vi "park snom main.vi"() -> ()   [LabVIEW 2021]
panel:
  in  "Comments 3":string
  in  "Comments 2":string
  in  "Comments 1":string
  in  "Load Pos 3":bool
  in  "Load Pos 2":bool
  in  "Load Pos 1":bool
  in  "Save Position 3":bool
  in  "Save Position 2":bool
  out "Position 3":T1
  out "Position 2":T1
  out "Position 1":T1
  in  "Time To Wait":dbl
  out "Scan Origin (ALS)":T1
  in  "minimum value":dbl=-5.0 format="%0.2f"
  in  "maximum value":dbl=5.0 format="%0.2f"
  in  "Read pos on/off":bool
  in  "Save Waveform Graph":bool
  in  "Update\nphi/theta":bool
  in  "dz":dbl
  in  "dy":dbl
  in  "dx":dbl
  in  "Move to rho":bool
  out "Current Volts":dbl format="%0.7f"
  out "Waveform Graph":dbl[](graph)
  in  "Angeled Line\nScan":bool
  in  "rho Step Size (microns)":dbl=10.0
  in  "rho Length (microns)":dbl=1000.0
  in  "phi":dbl
  in  "theta":dbl
  in  "Z":string="3"
  in  "Y":string="2"
  in  "X":string="1"
  in  "First Time?":bool
  in  "Save Position 1":bool
  out "Estimated\nTime Left":dbl
  out "Percent Complete":dbl
  in  "Back scan delay":u32
  in  "Angled Scan":bool
  in  "Angle":dbl
  out "Scan Type":string="Start Point Serpent Scan"
  in  "T=SP \nf=CP":bool
  in  "Save Intensity Graph":bool
  in  "Export Data to Excel":bool
  in  "Center Typewritter\nScan":bool
  in  "Center Serpent\nScan":bool
  out "Measured":dbl
  out "Absolute 1 time":u32
  in  "physical channels":tag="Dev1/ai7"
  out "Time per Pixel":u32
  in  "Command":string
  in  "Controller #":string
  in  "Command":bool
  out "Graph":dbl[][](graph)
  in  "rate":dbl=250000.0
  in  "number of samples":i32=100
  out "Slow Axis Pos\n(Max)":dbl
  out "Fast Axis Pos\n(Max)":dbl
  out "Min Value":dbl
  in  "Move to Max\nValue Position":bool
  out "Max Value":dbl
  in  "Move to Cursor 2":bool
  in  "Move to Cursor 1":bool
  out "Scan Origin":T1
  in  "Move 3 By":dbl=1.0
  in  "Move 2 By":dbl=1.0
  in  "Move 3 to":dbl=12.0
  in  "Move 2 to":dbl=3.8
  in  "PL 3":dbl=22.2
  in  "PL 2":dbl=12.2
  in  "PL 1":dbl=12.2
  in  "NL 3":dbl
  in  "NL 2":dbl
  in  "NL 1":dbl
  in  "Set Limits":bool
  in  "Move All":bool
  in  "Update Params":bool
  in  "Start Point\nTypewriter Scan":bool
  in  "Initialize?":bool
  in  "Abort Scan":bool
  in  "Start Point\nSerpent Scan":bool
  in  "Slow Length (microns)":dbl=500.0
  in  "Slow Step Size (microns)":dbl=100.0
  in  "Fast Length (microns)":dbl=500.0
  in  "Fast Step Size (microns)":dbl=100.0
  in  "Slow Axis":string="3"
  in  "Fast Axis":string="1"
  in  "Update Loop Type":bool
  in  "Loop Type":string="2"
  in  "Motion Parameters In":T2={"Velocity"=2.0, "Deceleration "=100.0, "Acceleration"=100.0}
  out "Motion Parameters Out":T3={"Velocity "=2.0, "Deceleration "=100.0, "Acceleration"=100.0}
  out "Calculated Position":T1
  out "Encoder Position":T4
  in  "Move 1 to":dbl=6.0
  in  "Move 1 By":dbl=1.0
  in  "Motor 3":bool
  in  "Motor 2":bool
  in  "< 3":bool
  in  "> 3":bool
  in  "< 2":bool
  in  "> 2":bool
  in  "<":bool
  in  ">":bool
  in  "Motor 1":bool
  in  "End":bool
  # "Positioning"
  # "Motion Parameters"
  # "mm/s"
  # "mm"
  # "mm"
  # "Controller #1"
  # "mm"
  # "mm/s^2"
  # "Controller #2"
  # "mm"
  # "mm"
  # "mm/s^2"
  # "Controller #3"
  # "mm"
  # "mm"
  # "mm"
  # "V"
  # "msec"
  # "Motor 1"
  # "mm"
  # "mm"
  # "min"
  # "Motor 2"
  # "0: Open Loop\n2: Clean Closed Loop\n3: Closed Loop"
  # "mm"
  # "mm"
  # "Motor 3"
  # "mm"
  # "mm"
  # "mm"
  # "mm"
  # "mm"
  # "mm"
  # "Might have to\npress twice"
  # "mm"
  # "mm"
  # "mm"
  # "mm"
  # "mm"
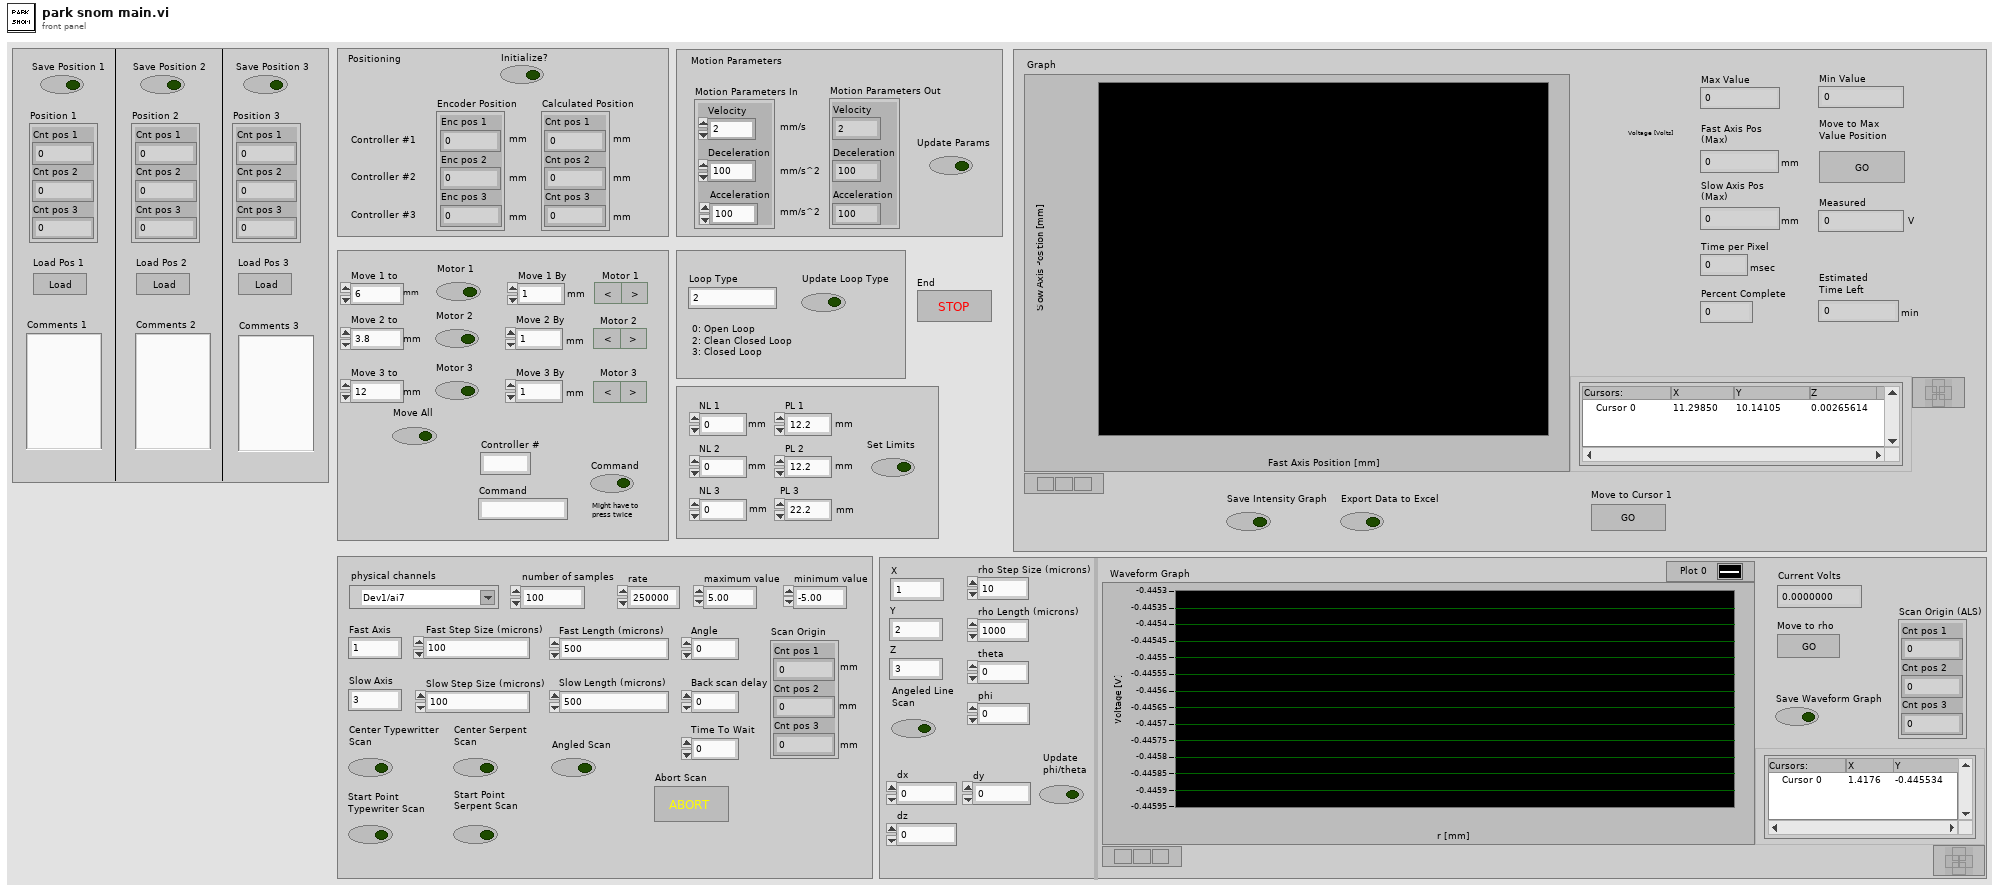
[diagram p1: front panel]
types:
  T1 = cluster{"Cnt pos 1":dbl, "Cnt pos 2":dbl, "Cnt pos 3":dbl}
  T2 = cluster{"Velocity":dbl, "Deceleration ":dbl, "Acceleration":dbl}
  T3 = cluster{"Velocity ":dbl, "Deceleration ":dbl, "Acceleration":dbl}
  T4 = cluster{"Enc pos 1":dbl, "Enc pos 2":dbl, "Enc pos 3":dbl}
  T5 = cluster{"P type":u16, "VISA resource name out":refnum<visa-resource-name>, " Terminator":string, "Timeout":i32}
  T6 = cluster{"P type":u16, "reference":refnum<visa-resource-name>, " Terminator ":string, "Timeout":i32}
  T7 = typedef "LVPointDoubleTypeDef.ctl" = cluster{"Cursor X":dbl, "Cursor Y":dbl}
  T8 = typedef "LVCursorListTypeDef.ctl" = cluster{"Name":string, "Color":u32, "Style":u8, "Point Style":u8, "Name Visible":bool, "Allow Drag":bool, "Cursor Mode":u32, "Plot":i32, "Index":i32, "Position":cluster{"X":dbl, "Y":dbl}, "X Scale":u32, "Y Scale":u32, "Watch Plots":i32[], "Watch All Plots":bool, "Plot Area":i32, "Label Offset":cluster{"X":dbl, "Y":dbl}}[]
  T9 = typedef "imagedata.ctl" = cluster{"image type":i32, "image depth":i32, "image":u8[], "mask":u8[], "colors":u32[], "Rectangle":cluster{"left":i16, "top":i16, "right":i16, "bottom":i16}}
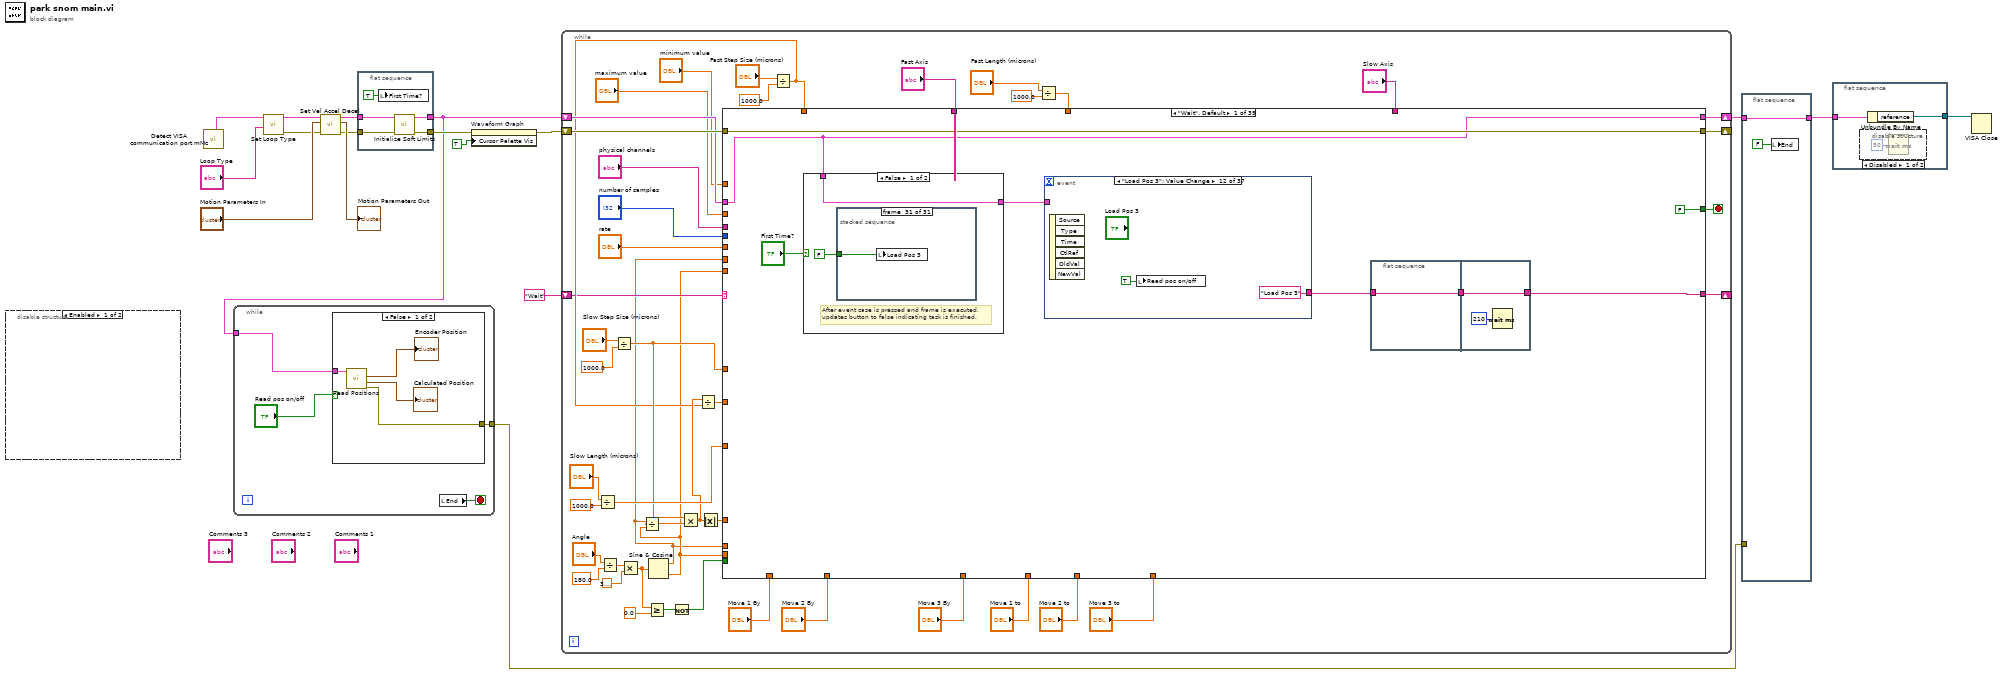
[diagram p0: block diagram]
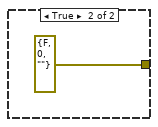
[diagram p2: hidden frame]
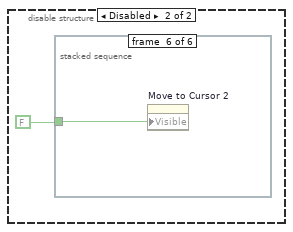
[diagram p3: hidden frame]
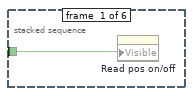
[diagram p4: hidden frame]
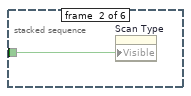
[diagram p5: hidden frame]
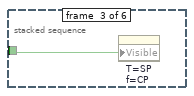
[diagram p6: hidden frame]
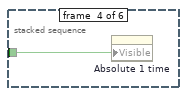
[diagram p7: hidden frame]
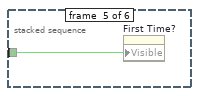
[diagram p8: hidden frame]
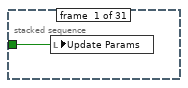
[diagram p10: hidden frame]
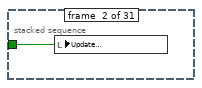
[diagram p11: hidden frame]
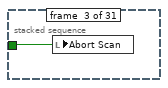
[diagram p12: hidden frame]
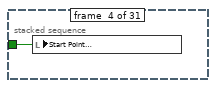
[diagram p13: hidden frame]
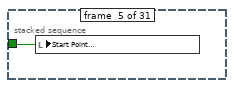
[diagram p14: hidden frame]
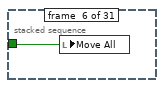
[diagram p15: hidden frame]
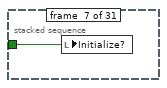
[diagram p16: hidden frame]
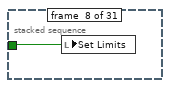
[diagram p17: hidden frame]
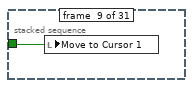
[diagram p18: hidden frame]
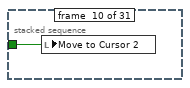
[diagram p19: hidden frame]
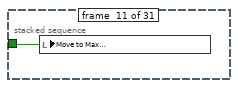
[diagram p20: hidden frame]
diagram:
  n1 = disable-structure shown="Enabled" {
    frame Enabled {
    }
    frame Disabled {
      n2 = stacked-sequence {
        tunnel: FALSE -> [w19 w20 w21 w22 w23 w24]
        frame #0 {
          n3 = property on="Read pos on/off" class="Bool (strict)"("Visible"=w19) -> ()  [unwired: 2 in, 2 out]
        }
        frame #1 {
          n4 = property on="Scan Type" class="Str"("Visible"=w20) -> ()  [unwired: 2 in, 2 out]
        }
        frame #2 {
          n5 = property on="T=SP \nf=CP" class="Bool (strict)"("Visible"=w21) -> ()  [unwired: 2 in, 2 out]
        }
        frame #3 {
          n6 = property on="Absolute 1 time" class="DigNum (strict)"("Visible"=w22) -> ()  [unwired: 2 in, 2 out]
        }
        frame #4 {
          n7 = property on="First Time?" class="Bool (strict)"("Visible"=w23) -> ()  [unwired: 2 in, 2 out]
        }
        frame #5 {
          n8 = property on="Move to Cursor 2" class="Bool (strict)"("Visible"=w24) -> ()  [unwired: 2 in, 2 out]
        }
      }
    }
  }
  n9 = call "Detect VISA communication port mMc.vi"() -> ("Port"=w14:T5)  [unwired: 6 in, 3 out]
  n10 = while {
    tunnel: w1 -> [w26]
    tunnel: [w27] -> w8
    stop <- w28 stop-if-true
    n11 = case shown="False" "Read pos on/off" {
      tunnel: [w30 errorcluster {"status"=FALSE, "code"=0, "source"=""} ("error out")] -> w27
      tunnel: w26 -> [w29 _]
      frame False {
        n12 = call "Read Positions.vi"("Port In"=w29) -> ("error out"=w30:errorcluster, "Calculated Position"=→"Calculated Position":T1, "Encoder Position"=→"Encoder Position":T4)  [unwired: 7 in, 1 out]
      }
      frame True {
      }
    }
    n13 = local read "End"() -> (w28:bool)
  }
  n14 = call "Set Loop Type.vi"("Loop Type"="Loop Type", "Port In"=w14) -> ("error out"=w5:errorcluster, "Port Out"=w12:T5)  [unwired: 8 in]
  n15 = call "Set Vel Accel Decel.vi"("error in (no error)"=w5, "Motion Parameters In"="Motion Parameters In", "Port In"=w12) -> ("error out"=w6:errorcluster, "Motion Parameters Out"=→"Motion Parameters Out":T3, "Port Out"=w7:T5)  [unwired: 6 in]
  n16 = flat-sequence {
    tunnel: w7 -> [w38]
    tunnel: w6 -> [w37]
    tunnel: [w36] -> w1
    tunnel: [w35] -> w3
    frame #0 {
      n17 = local write "First Time?"(TRUE ("first time")) -> ()
      n18 = call "Initialize Soft Limits.vi"("error in (no error)"=w37, "Port In"=w38) -> ("error out"=w35:errorcluster, "Port Out"=w36:T6)  [unwired: 8 in]
    }
  }
  n19 = property on="Waveform Graph" class="WFGraph (strict)"(error in=w3, "Cursor Palette Vis"=TRUE ("Cursor Legend Visible")) -> (error out=w2:errorcluster)  [unwired: 1 in, 1 out]
  n20 = while {
    shift-right: [w84] -> _
    shift-left: "Wait" -> [w48]
    shift-right: [w80] -> _
    shift-left: w2 -> [w83]
    shift-right: [w79] -> w10
    shift-left: w1 -> [w68]
    stop <- w81 stop-if-true
    n21 = Divide(x="Slow Length (microns)", y=1000.0) -> (x/y=w54:dbl)
    n22 = Divide(x="Angle", y=180.0) -> (x/y=w56:dbl)
    n23 = Divide(x="Slow Step Size (microns)", y=1000.0) -> (x/y=w51:dbl)
    n24 = Multiply(x=w56, y=3.141592653589793) -> (x*y=w44:dbl)
    n25 = Greater Or Equal?(x=w44, y=0.0) -> (x >= y?=w46:bool)
    n26 = Sine & Cosine(0:w44) -> (1:w41:dbl, 2:w42:dbl)
    n27 = Divide(x=w41, y=w42) -> (x/y=w43:dbl)
    n28 = Not(x=w46) -> (.not. x?=w45:bool)
    n29 = Multiply(x=w51, y=w43) -> (x*y=w50:dbl)
    n30 = Absolute Value(x=w50) -> (abs(x)=w53:dbl)
    n31 = Divide(x="Fast Step Size (microns)", y=1000.0) -> (x/y=w49:dbl)
    n32 = Divide(x=w50, y=w49) -> (x/y=w47:dbl)
    n33 = Divide(x="Fast Length (microns)", y=1000.0) -> (x/y=w60:dbl)
    n34 = case shown="\"Wait\", Default" w48 {
      tunnel: [w89 "Stop" "Update Limits" "Wait" "Wait" "Wait" "Wait" ("Scan Type") "Wait" ("Scan Type") "Wait" ("Scan Type") "Wait" ("Scan Type") "Wait" ("Scan Type") "Wait" ("Scan Type") "Wait" ("Scan Type") "Wait" "Wait" "Wait" "Wait" "Wait" "Wait" "Wait" "Wait" "Wait" "Wait" "Wait" w481 "Move to Origin" "Move to Origin" "Move to Origin" "Move to Origin" "Move to Origin" w1566 "Wait" "Wait" "Wait" "Wait" "Wait" ("Scan Type") "Wait" "Wait" "Wait"] -> w84
      tunnel: "Move 1 to" -> [_ _ _ _ _ _ _ _ _ _ _ _ _ w334 _ _ w384 _ _ _ _ _ _ _ _ _ _ _ _ _ _ _ _ _ _ _ _ _ _]
      tunnel: w68 -> [w85 w209 w218 w236 w248 w259 w264 w272 w277 w281 w289 w297 w315 w333 w359 w367 w379 w393 w411 w420 w429 w438 w447 w462 w483 w542 w732 w929 w1107 w1312 w1565 w1686 w1706 w1728 w1745 w1775 w1834 w1839 w1846]
      tunnel: w83 -> [w92 w211 w221 w235 w247 w257 w263 w271 w276 w282 w290 w298 w316 w342 w363 w371 w389 w397 w416 w425 w434 w443 w452 w463 w482 w552 w752 w940 w1140 w1341 w1592 w1683 w1703 w1723 w1740 w1782 w1837 w1840 w1847]
      tunnel: [w92 w211 w221 w233 w247 w257 w263 w271 w276 w282 w290 w298 w316 w342 w363 w371 w389 w397 w416 w425 w434 w443 w452 w463 w482 w552 w752 w940 w1140 w1341 w1592 w1683 w1703 w1723 w1740 w1782 w1837 w1840 w1847] -> w80
      tunnel: [FALSE TRUE FALSE FALSE FALSE FALSE FALSE FALSE FALSE FALSE FALSE FALSE FALSE FALSE FALSE FALSE FALSE FALSE FALSE FALSE FALSE FALSE FALSE FALSE FALSE FALSE FALSE FALSE FALSE FALSE FALSE FALSE FALSE FALSE FALSE FALSE FALSE FALSE FALSE] -> w81
      tunnel: [w85 w209 w222 w232 w244 w258 w264 w272 w277 w281 w289 w297 w315 w340 w357 w365 w373 w391 w409 w418 w427 w436 w445 w462 w483 w542 w732 w929 w1107 w1312 w1593 w1679 w1699 w1720 w1737 w1775 w1827 w1839 w1846] -> w79
      tunnel: w51 -> [_ _ _ _ _ _ _ _ _ _ _ _ _ _ _ _ _ _ _ _ _ _ _ _ w495 w546 w748 w935 w1136 w1337 _ _ _ _ _ _ _ _ _]
      tunnel: w54 -> [_ _ _ _ _ _ _ _ _ _ _ _ _ _ _ _ _ _ _ _ _ _ _ _ w485 w547 w738 w924 w1125 w1326 _ _ _ _ _ _ _ _ _]
      tunnel: w49 -> [_ _ _ _ _ _ _ _ _ _ _ _ _ _ _ _ _ _ _ _ _ _ _ _ w496 w531 w717 w920 w1100 w1311 _ _ _ _ _ _ _ _ _]
      tunnel: w60 -> [_ _ _ _ _ _ _ _ _ _ _ _ _ _ _ _ _ _ _ _ _ _ _ _ w493 w534 w719 w921 w1109 w1313 _ _ _ _ _ _ _ _ _]
      tunnel: "Fast Axis" -> [_ _ _ _ _ _ _ _ _ _ _ _ _ _ _ _ _ _ _ _ _ _ _ _ w494 w538 w726 w938 w1116 w1306 _ _ _ w1727 w1744 _ w1833 _ _]
      tunnel: "Slow Axis" -> [_ _ _ _ _ _ _ _ _ _ _ _ _ _ _ _ _ _ _ _ _ _ _ _ w486 w550 w730 w931 w1106 w1309 _ _ _ w1726 w1743 _ w1832 _ _]
      tunnel: "Move 2 to" -> [_ _ _ _ _ _ _ _ _ _ _ _ _ _ w358 _ w383 _ _ _ _ _ _ _ _ _ _ _ _ _ _ _ _ _ _ _ _ _ _]
      tunnel: "Move 3 to" -> [_ _ _ _ _ _ _ _ _ _ _ _ _ _ _ w366 w382 _ _ _ _ _ _ _ _ _ _ _ _ _ _ _ _ _ _ _ _ _ _]
      tunnel: "Move 1 By" -> [_ _ _ _ _ _ _ _ _ _ _ _ _ _ _ _ _ w392 _ _ w428 _ _ _ _ _ _ _ _ _ _ _ _ _ _ _ _ _ _]
      tunnel: "Move 2 By" -> [_ _ _ _ _ _ _ _ _ _ _ _ _ _ _ _ _ _ w410 _ _ w437 _ _ _ _ _ _ _ _ _ _ _ _ _ _ _ _ _]
      tunnel: "Move 3 By" -> [_ _ _ _ _ _ _ _ _ _ _ _ _ _ _ _ _ _ _ w419 _ _ w446 _ _ _ _ _ _ _ _ _ _ _ _ _ _ _ _]
      tunnel: "number of samples" -> [_ _ _ _ _ _ _ _ _ _ _ _ _ _ _ _ _ _ _ _ _ _ _ _ _ w537 w740 w925 w1128 w1329 w1568 _ _ _ _ _ _ _ _]
      tunnel: "rate" -> [_ _ _ _ _ _ _ _ _ _ _ _ _ _ _ _ _ _ _ _ _ _ _ _ _ w540 w742 w928 w1131 w1332 w1589 _ _ _ _ _ _ _ _]
      tunnel: "physical channels" -> [_ _ _ _ _ _ _ _ _ _ _ _ _ _ _ _ _ _ _ _ _ _ _ _ _ w539 w741 w926 w1129 w1330 w1590 _ _ _ _ _ _ _ _]
      tunnel: w53 -> [_ _ _ _ _ _ _ _ _ _ _ _ _ _ _ _ _ _ _ _ _ _ _ _ _ w532 w718 w919 w1101 _ _ _ _ _ _ _ _ _ _]
      tunnel: w45 -> [_ _ _ _ _ _ _ _ _ _ _ _ _ _ _ _ _ _ _ _ _ _ _ _ _ w535 w721 w922 w1111 _ _ _ _ _ _ _ _ _ _]
      tunnel: w47 -> [_ _ _ _ _ _ _ _ _ _ _ _ _ _ _ _ _ _ _ _ _ _ _ _ _ w525 w711 w913 w1110 _ _ _ _ _ _ _ _ _ _]
      tunnel: w42 -> [_ _ _ _ _ _ _ _ _ _ _ _ _ _ _ _ _ _ _ _ _ _ _ _ _ _ _ _ _ w1308 _ _ _ _ _ _ _ _ _]
      tunnel: w41 -> [_ _ _ _ _ _ _ _ _ _ _ _ _ _ _ _ _ _ _ _ _ _ _ _ _ _ _ _ _ w1307 _ _ _ _ _ _ _ _ _]
      tunnel: w42 -> [_ _ _ _ _ _ _ _ _ _ _ _ _ _ _ _ _ _ _ _ _ _ _ _ _ _ _ _ _ w1305 _ _ _ _ _ _ _ _ _]
      tunnel: w41 -> [_ _ _ _ _ _ _ _ _ _ _ _ _ _ _ _ _ _ _ _ _ _ _ _ _ _ _ _ _ w1304 _ _ _ _ _ _ _ _ _]
      tunnel: "maximum value" -> [_ _ _ _ _ _ _ _ _ _ _ _ _ _ _ _ _ _ _ _ _ _ _ _ _ w522 w709 w910 w1097 w1301 w1539 _ _ _ _ _ _ _ _]
      tunnel: "minimum value" -> [_ _ _ _ _ _ _ _ _ _ _ _ _ _ _ _ _ _ _ _ _ _ _ _ _ w521 w708 w909 w1096 w1300 w1538 _ _ _ _ _ _ _ _]
      frame "Wait", Default {
        n35 = case shown="False" "First Time?" {
          tunnel: [w93 w126] -> w86
          tunnel: w85 -> [w93 w126]
          frame False {
            # "After event case is pressed and frame is executed, \nupdates button to false indicating task is finished."
            n36 = stacked-sequence {
              tunnel: FALSE ("Command") -> [w95 w96 w97 w98 w99 w100 w101 w102 w103 w104 w105 w106 w107 w108 w109 w110 w111 w112 w113 w114 w115 w116 w117 w118 w119 w120 w121 w122 w123 w124 w125]
              frame #0 {
                n37 = local write "Update Params"(w95) -> ()
              }
              frame #1 {
                n38 = local write "Update\nphi/theta"(w96) -> ()
              }
              frame #2 {
                n39 = local write "Abort Scan"(w97) -> ()
              }
              frame #3 {
                n40 = local write "Start Point\nSerpent Scan"(w98) -> ()
              }
              frame #4 {
                n41 = local write "Start Point\nTypewriter Scan"(w99) -> ()
              }
              frame #5 {
                n42 = local write "Move All"(w100) -> ()
              }
              frame #6 {
                n43 = local write "Initialize?"(w101) -> ()
              }
              frame #7 {
                n44 = local write "Set Limits"(w102) -> ()
              }
              frame #8 {
                n45 = local write "Move to Cursor 1"(w103) -> ()
              }
              frame #9 {
                n46 = local write "Move to Cursor 2"(w104) -> ()
              }
              frame #10 {
                n47 = local write "Move to Max\nValue Position"(w105) -> ()
              }
              frame #11 {
                n48 = local write "Motor 1"(w106) -> ()
              }
              frame #12 {
                n49 = local write "Motor 2"(w107) -> ()
              }
              frame #13 {
                n50 = local write "Motor 3"(w108) -> ()
              }
              frame #14 {
                n51 = local write "Command"(w109) -> ()
              }
              frame #15 {
                n52 = local write "Center Serpent\nScan"(w110) -> ()
              }
              frame #16 {
                n53 = local write "Center Typewritter\nScan"(w111) -> ()
              }
              frame #17 {
                n54 = local write "Export Data to Excel"(w112) -> ()
              }
              frame #18 {
                n55 = local write "Save Intensity Graph"(w113) -> ()
              }
              frame #19 {
                n56 = local write "Angled Scan"(w114) -> ()
              }
              frame #20 {
                n57 = local write "Save Position 1"(w115) -> ()
              }
              frame #21 {
                n58 = local write "Angeled Line\nScan"(w116) -> ()
              }
              frame #22 {
                n59 = local write "Move to rho"(w117) -> ()
              }
              frame #23 {
                n60 = local write "Save Waveform Graph"(w118) -> ()
              }
              frame #24 {
                n61 = local write "Read pos on/off"(w119) -> ()
              }
              frame #25 {
                n62 = local write "Save Position 1"(w120) -> ()
              }
              frame #26 {
                n63 = local write "Save Position 2"(w121) -> ()
              }
              frame #27 {
                n64 = local write "Save Position 3"(w122) -> ()
              }
              frame #28 {
                n65 = local write "Load Pos 1"(w123) -> ()
              }
              frame #29 {
                n66 = local write "Load Pos 2"(w124) -> ()
              }
              frame #30 {
                n67 = local write "Load Pos 3"(w125) -> ()
              }
            }
          }
          frame True {
            n68 = local write "First Time?"(FALSE ("first time")) -> ()
          }
        }
        n69 = event shown="[11] \"Load Pos 3\": Value Change" {
          selector: _ -> [_ _ _ _ _ _ _ _ _ _ _ _ _ _ _ _ _ _ _ _ _ _ _ _ _ _ _ _ _ _ _ _ _ _ _ _ _]
          dyn-events: _ -> [_ _ _ _ _ _ _ _ _ _ _ _ _ _ _ _ _ _ _ _ _ _ _ _ _ _ _ _ _ _ _ _ _ _ _ _ _]
          timeout: _ -> [_ _ _ _ _ _ _ _ _ _ _ _ _ _ _ _ _ _ _ _ _ _ _ _ _ _ _ _ _ _ _ _ _ _ _ _ _]
          tunnel: ["Wait" "Stop" "Initialize" "Move Command" "Update Loop Type" "Update Params" "Save Position 1" "Save Position 2" "Save Position 3" "Load Pos 1" "Load Pos 2" "Load Pos 3" "Update phi/theta" "Motor 1 Absolute" "Motor 2 Absolute" "Motor 3 Absolute" "All Motors Absolute" "Motor 1 Positive Relative" "Motor 1 Negative Relative" "Motor 2 Positive Relative" "Motor 2 Negative Relative" "Motor 3 Positive Relative" "Motor 3 Negative Relative" "Update Limits" "Initialize Graph" "Initialize Graph" "Initialize Graph" "Initialize Graph" "Initialize Graph" "Angeled Line Scan" "Move to Cursor 1" "Move to Cursor 2" "Move to rho" "Move to Max Value Position" "Export Data" "Save Image" "Save Image"] -> w91
          tunnel: w86 -> [_ _ _ _ _ _ _ _ _ _ _ _ _ _ _ _ _ _ _ _ _ _ _ _ w169 w179 w182 w191 w197 w200 _ _ _ _ _ _ _]
          event Timeout {
            n70 = event-data() -> ()  [unwired: 1 in, 3 out]
          }
          event "End": Value Change {
            n71 = event-data() -> ()  [unwired: 1 in, 6 out]
          }
          event "Initialize?": Value Change {
            n72 = event-data() -> ()  [unwired: 1 in, 6 out]
          }
          event "Command": Value Change {
            n73 = event-data() -> ()  [unwired: 1 in, 6 out]
            n74 = local write "Command"(TRUE ("Command")) -> ()
          }
          event "Update Loop Type": Value Change {
            n75 = event-data() -> ()  [unwired: 1 in, 6 out]
          }
          event "Update Params": Value Change {
            n76 = event-data() -> ()  [unwired: 1 in, 6 out]
          }
          event "Save Position 1": Value Change {
            n77 = event-data() -> ()  [unwired: 1 in, 6 out]
            n78 = local write "Read pos on/off"(TRUE ("Save Position")) -> ()
          }
          event "Save Position 2": Value Change {
            n79 = event-data() -> ()  [unwired: 1 in, 6 out]
            n80 = local write "Read pos on/off"(TRUE ("Read pos on/off")) -> ()
          }
          event "Save Position 3": Value Change {
            n81 = event-data() -> ()  [unwired: 1 in, 6 out]
            n82 = local write "Read pos on/off"(TRUE ("Read pos on/off")) -> ()
          }
          event "Load Pos 1": Value Change {
            n83 = event-data() -> ()  [unwired: 1 in, 6 out]
            n84 = local write "Read pos on/off"(TRUE ("Read pos on/off")) -> ()
          }
          event "Load Pos 2": Value Change {
            n85 = event-data() -> ()  [unwired: 1 in, 6 out]
            n86 = local write "Read pos on/off"(TRUE ("Read pos on/off")) -> ()
          }
          event "Load Pos 3": Value Change {
            n87 = event-data() -> ()  [unwired: 1 in, 6 out]
            n88 = local write "Read pos on/off"(TRUE ("Read pos on/off")) -> ()
          }
          event "Update\nphi/theta": Value Change {
            n89 = event-data() -> ()  [unwired: 1 in, 6 out]
          }
          event "Motor 1": Value Change {
            n90 = event-data() -> ()  [unwired: 1 in, 6 out]
          }
          event "Motor 2": Value Change {
            n91 = event-data() -> ()  [unwired: 1 in, 6 out]
          }
          event "Motor 3": Value Change {
            n92 = event-data() -> ()  [unwired: 1 in, 6 out]
          }
          event "Move All": Value Change {
            n93 = event-data() -> ()  [unwired: 1 in, 6 out]
          }
          event ">": Value Change {
            n94 = event-data() -> ()  [unwired: 1 in, 6 out]
            n95 = local write "Read pos on/off"(TRUE ("Read pos on/off")) -> ()
          }
          event "<": Value Change {
            n96 = event-data() -> ()  [unwired: 1 in, 6 out]
            n97 = local write "Read pos on/off"(TRUE) -> ()
          }
          event "> 2": Value Change {
            n98 = event-data() -> ()  [unwired: 1 in, 6 out]
            n99 = local write "Read pos on/off"(TRUE) -> ()
          }
          event "< 2": Value Change {
            n100 = event-data() -> ()  [unwired: 1 in, 6 out]
            n101 = local write "Read pos on/off"(TRUE) -> ()
          }
          event "> 3": Value Change {
            n102 = event-data() -> ()  [unwired: 1 in, 6 out]
            n103 = local write "Read pos on/off"(TRUE) -> ()
          }
          event "< 3": Value Change {
            n104 = event-data() -> ()  [unwired: 1 in, 6 out]
            n105 = local write "Read pos on/off"(TRUE) -> ()
          }
          event "Set Limits": Value Change {
            n106 = event-data() -> ()  [unwired: 1 in, 6 out]
          }
          event "Start Point\nSerpent Scan": Value Change {
            n107 = event-data() -> ()  [unwired: 1 in, 6 out]
            n108 = local write "Read pos on/off"(TRUE ("Read pos on/off")) -> ()
            n109 = call "Read Positions.vi"("Port In"=w169) -> ("Calculated Position"=w173:T1)  [unwired: 7 in, 3 out]
            n110 = local write "Scan Origin"(w173) -> ()
            n111 = local write "T=SP \nf=CP"(TRUE ("T=SP \nf=CP")) -> ()
            "Scan Type" <- "Start Point Serpent Scan"
          }
          event "Center Serpent\nScan": Value Change {
            n112 = event-data() -> ()  [unwired: 1 in, 6 out]
            n113 = local write "Read pos on/off"(TRUE ("Read pos on/off")) -> ()
            n114 = local write "Scan Type"("Center Serpent Scan") -> ()
            n115 = call "Read Positions.vi"("Port In"=w179) -> ("Calculated Position"=w174:T1)  [unwired: 7 in, 3 out]
            n116 = local write "Scan Origin"(w174) -> ()
            n117 = local write "T=SP \nf=CP"(FALSE ("T=SP \nf=CP")) -> ()
          }
          event "Start Point\nTypewriter Scan": Value Change {
            n118 = event-data() -> ()  [unwired: 1 in, 6 out]
            n119 = local write "Read pos on/off"(TRUE ("Read pos on/off")) -> ()
            n120 = call "Read Positions.vi"("Port In"=w182) -> ("Calculated Position"=w185:T1)  [unwired: 7 in, 3 out]
            n121 = local write "Scan Type"("Start Point Typewriter Scan") -> ()
            n122 = local write "T=SP \nf=CP"(TRUE ("Status Bit")) -> ()
            n123 = local write "Scan Origin"(w185) -> ()
          }
          event "Center Typewritter\nScan": Value Change {
            n124 = event-data() -> ()  [unwired: 1 in, 6 out]
            n125 = local write "Read pos on/off"(TRUE ("Read pos on/off")) -> ()
            n126 = local write "Scan Type"("Center Typewriter Scan") -> ()
            n127 = call "Read Positions.vi"("Port In"=w191) -> ("Calculated Position"=w190:T1)  [unwired: 7 in, 3 out]
            n128 = local write "Scan Origin"(w190) -> ()
            n129 = local write "T=SP \nf=CP"(FALSE ("T=SP \nf=CP")) -> ()
          }
          event "Angled Scan": Value Change {
            n130 = event-data() -> ()  [unwired: 1 in, 6 out]
            n131 = local write "Read pos on/off"(TRUE ("Read pos on/off")) -> ()
            n132 = local write "Scan Type"("Angeled Scan") -> ()
            n133 = call "Read Positions.vi"("Port In"=w197) -> ("Calculated Position"=w196:T1)  [unwired: 7 in, 3 out]
            n134 = local write "Scan Origin"(w196) -> ()
            n135 = local write "T=SP \nf=CP"(FALSE ("T=SP \nf=CP")) -> ()
          }
          event "Angeled Line\nScan": Value Change {
            n136 = event-data() -> ()  [unwired: 1 in, 6 out]
            n137 = local write "Read pos on/off"(TRUE ("Read pos on/off")) -> ()
            n138 = call "Read Positions.vi"("Port In"=w200) -> ("Calculated Position"=→"Scan Origin (ALS)":T1)  [unwired: 7 in, 3 out]
          }
          event "Move to Cursor 1": Value Change {
            n139 = event-data() -> ()  [unwired: 1 in, 6 out]
          }
          event "Move to Cursor 2": Value Change {
            n140 = event-data() -> ()  [unwired: 1 in, 6 out]
          }
          event "Move to rho": Value Change {
            n141 = event-data() -> ()  [unwired: 1 in, 6 out]
          }
          event "Move to Max\nValue Position": Value Change {
            n142 = event-data() -> ()  [unwired: 1 in, 6 out]
          }
          event "Export Data to Excel": Value Change {
            n143 = event-data() -> ()  [unwired: 1 in, 6 out]
          }
          event "Save Intensity Graph": Value Change {
            n144 = event-data() -> ()  [unwired: 1 in, 6 out]
          }
          event "Save Waveform Graph": Value Change {
            n145 = event-data() -> ()  [unwired: 1 in, 6 out]
          }
        }
        n146 = flat-sequence {
          tunnel: w91 -> [w128]
          tunnel: [w128] -> w88
          tunnel: [w130] -> w89
          tunnel: w88 -> [w130]
          frame #0 {
          }
          frame #1 {
            n147 = Wait (ms)(milliseconds to wait=u32 210) -> ()  [unwired: 1 out]
          }
        }
      }
      frame "Stop" {
        n148 = Wait (ms)(milliseconds to wait=u32 50) -> ()  [unwired: 1 out]
      }
      frame "Initialize" {
        # "Moves to the negative limit of each motor\nand zeros the position at that location"
        # "Prevents overwriting the VISA"
        # "Sets the range of motion (limit) of each motor to -999 and 999, respectively"
        n149 = call "Initialize Soft Limits.vi"("Port In"=w218) -> ("error out"=w215:errorcluster, "Port Out"=w216:T6)  [unwired: 9 in]
        n150 = flat-sequence {
          tunnel: [w225] -> w217
          tunnel: w216 -> [w225]
          tunnel: w215 -> [w224]
          tunnel: [w224] -> w214
          frame #0 {
            n151 = Wait (ms)(milliseconds to wait=u32 30) -> ()  [unwired: 1 out]
          }
        }
        n152 = call "Initialize Axes.vi"("error in (no error)"=w214, "Port In"=w217) -> ("Port Out"=w222:T5)  [unwired: 8 in, 1 out]
      }
      frame "Move Command" {
        # "Gives a command to a controller"
        n153 = call "Give Move Command.vi"("error in (no error)"=w235, "Command"="Command", "Port In"=w236, "Controller #"="Controller #") -> ("error out"=w230:errorcluster, "Port Out"=w231:T5)  [unwired: 6 in]
        n154 = flat-sequence {
          tunnel: w231 -> [w240]
          tunnel: w230 -> [w241]
          tunnel: [w241] -> w229
          tunnel: [w240] -> w228
          tunnel: "Controller #" -> [w239]
          tunnel: [w239] -> w226
          frame #0 {
            n155 = Wait (ms)(milliseconds to wait=u32 30) -> ()  [unwired: 1 out]
          }
        }
        n156 = call "Check Idle (non scan).vi"("error in (no error)"=w229, "Controller #"=w226, "Port In"=w228) -> ("error out (no error)"=w233:errorcluster, "Port Out"=w232:T6)  [unwired: 7 in]
      }
      frame "Update Loop Type" {
        n157 = flat-sequence {
          tunnel: w248 -> [w251]
          tunnel: [w249] -> w243
          tunnel: [w252] -> w244
          tunnel: w243 -> [w252]
          frame #0 {
            n158 = local read "Loop Type"() -> (w250:string)
            n159 = call "Set Loop Type.vi"("Loop Type"=w250, "Port In"=w251) -> ("Port Out"=w249:T5)  [unwired: 8 in, 1 out]
          }
          frame #1 {
            n160 = local write "Update Loop Type"(FALSE ("Update Loop Type")) -> ()
            n161 = Wait (ms)(milliseconds to wait=u32 100) -> ()  [unwired: 1 out]
          }
        }
      }
      frame "Update Params" {
        n162 = local read "Motion Parameters In"() -> (w260:T2)
        n163 = call "Set Vel Accel Decel.vi"("Motion Parameters In"=w260, "Port In"=w259) -> ("Motion Parameters Out"=w261:T3, "Port Out"=w258:T5)  [unwired: 7 in, 1 out]
        n164 = local write "Motion Parameters Out"(w261) -> ()
      }
      frame "Save Position 1" {
        n165 = disable-structure shown="Disabled" {
          frame Disabled {
            n166 = local read "Calculated Position"() -> (w270:T1)
            n167 = Unbundle By Name(w270) -> ("Cnt pos 1"=w269:dbl, "Cnt pos 2"=w268:dbl, "Cnt pos 3"=w267:dbl)
            n168 = local write "Move 1 to"(w269) -> ()
            n169 = local write "Move 2 to"(w268) -> ()
            n170 = local write "Move 3 to"(w267) -> ()
          }
          frame Enabled {
          }
        }
        n171 = local read "Calculated Position"() -> (→"Position 1":T1)
      }
      frame "Save Position 2" {
        n172 = local read "Calculated Position"() -> (→"Position 2":T1)
      }
      frame "Save Position 3" {
        n173 = local read "Calculated Position"() -> (→"Position 3":T1)
      }
      frame "Load Pos 1" {
        n174 = local read "Position 1"() -> (w288:T1)
        n175 = Unbundle By Name(w288) -> ("Cnt pos 1"=w287:dbl, "Cnt pos 2"=w286:dbl, "Cnt pos 3"=w285:dbl)
        n176 = local write "Move 2 to"(w286) -> ()
        n177 = local write "Move 1 to"(w287) -> ()
        n178 = local write "Move 3 to"(w285) -> ()
      }
      frame "Load Pos 2" {
        n179 = local read "Position 2"() -> (w296:T1)
        n180 = Unbundle By Name(w296) -> ("Cnt pos 1"=w295:dbl, "Cnt pos 2"=w294:dbl, "Cnt pos 3"=w293:dbl)
        n181 = local write "Move 1 to"(w295) -> ()
        n182 = local write "Move 2 to"(w294) -> ()
        n183 = local write "Move 3 to"(w293) -> ()
      }
      frame "Load Pos 3" {
        n184 = local read "Position 3"() -> (w304:T1)
        n185 = Unbundle By Name(w304) -> ("Cnt pos 1"=w303:dbl, "Cnt pos 2"=w302:dbl, "Cnt pos 3"=w301:dbl)
        n186 = local write "Move 1 to"(w303) -> ()
        n187 = local write "Move 2 to"(w302) -> ()
        n188 = local write "Move 3 to"(w301) -> ()
      }
      frame "Update phi/theta" {
        n189 = Divide(x="dy", y="dx") -> (x/y=w328:dbl)
        n190 = Inverse Tangent(1:w328) -> (0:w314:dbl)
        n191 = Divide(x=180.0, y=3.141592653589793) -> (x/y=w310:dbl)
        n192 = Square(x="dy") -> (x^2=w324:dbl)
        n193 = Square(x="dx") -> (x^2=w325:dbl)
        n194 = Square(x="dz") -> (x^2=w323:dbl)
        n195 = Multiply(x=w314, y=w310) -> (x*y=w313:dbl)
        n196 = local write "phi"(w313) -> ()
        n197 = Compound Arithmetic op=ADD(w325, w324, w323) -> (w322:dbl)
        n198 = Square Root(x=w322) -> (sqrt(x)=w320:dbl)
        n199 = Divide(x="dz", y=w320) -> (x/y=w319:dbl)
        n200 = Inverse Cosine(1:w319) -> (0:w308:dbl)
        n201 = Divide(x=180.0, y=3.141592653589793) -> (x/y=w306:dbl)
        n202 = Multiply(x=w308, y=w306) -> (x*y=w307:dbl)
        n203 = local write "theta"(w307) -> ()
      }
      frame "Motor 1 Absolute" {
        n204 = Tick Count (ms)() -> (millisecond timer value=w331:u32)
        n205 = disable-structure shown="Enabled" {
          disable-tunnel: [w348 w352] -> w335
          disable-tunnel: w334 -> [w347 w351]
          disable-tunnel: w333 -> [w346 w353]
          disable-tunnel: "1" ("Controller #") -> [w344 w349]
          disable-tunnel: w331 -> [w345 w350]
          disable-tunnel: [w345 w350] -> w330
          disable-tunnel: [w344 w349] -> w329
          frame Enabled {
            n206 = call "Move abs mMc.vi"("target pos in"=w347, "Port"=w346, "Controller #"=w344) -> ("error out"=w348:errorcluster)  [unwired: 6 in]
          }
          frame Disabled {
            n207 = call "Move abs mMc Edited.vi"("target pos in"=w351, "Controller #"=w349, "Port In"=w353) -> ("error out"=w352:errorcluster)  [unwired: 7 in, 1 out]
          }
        }
        n208 = flat-sequence {
          tunnel: [w356] -> w339
          tunnel: [w355] -> w338
          tunnel: [w354] -> w337
          tunnel: w335 -> [w356]
          tunnel: w330 -> [w354]
          frame #0 {
            n209 = Tick Count (ms)() -> (millisecond timer value=w355:u32)
          }
        }
        n210 = call "Check Idle (non scan).vi"("error in (no error)"=w339, "Controller #"=w329, "Port In"=w333) -> ("Port Out"=w340:T6)  [unwired: 7 in, 1 out]
        n211 = Subtract(x=w338, y=w337) -> (x-y=→"Absolute 1 time":u32)
      }
      frame "Motor 2 Absolute" {
        w360 = "2" ("Controller #")
        n212 = call "Move abs mMc.vi"("target pos in"=w358, "Port"=w359, "Controller #"=w360) -> ("error out"=w361:errorcluster)  [unwired: 6 in]
        n213 = call "Check Idle (non scan).vi"("error in (no error)"=w361, "Controller #"=w360, "Port In"=w359) -> ("Port Out"=w357:T6)  [unwired: 7 in, 1 out]
      }
      frame "Motor 3 Absolute" {
        w368 = "3" ("Controller #")
        n214 = call "Move abs mMc.vi"("target pos in"=w366, "Port"=w367, "Controller #"=w368) -> ("error out"=w369:errorcluster)  [unwired: 6 in]
        n215 = call "Check Idle (non scan).vi"("error in (no error)"=w369, "Controller #"=w368, "Port In"=w367) -> ("Port Out"=w365:T6)  [unwired: 7 in, 1 out]
      }
      frame "All Motors Absolute" {
        w385 = "3" ("Controller #")
        w377 = "2" ("Controller #")
        w378 = "1" ("Controller #")
        n216 = call "Move abs mMc.vi"("target pos in"=w384, "Port"=w379, "Controller #"=w378) -> ("error out"=w380:errorcluster)  [unwired: 6 in]
        n217 = call "Move abs mMc.vi"("target pos in"=w383, "Port"=w379, "error in (no error)"=w380, "Controller #"=w377) -> ("error out"=w381:errorcluster)  [unwired: 5 in]
        n218 = call "Move abs mMc.vi"("target pos in"=w382, "Port"=w379, "error in (no error)"=w381, "Controller #"=w385) -> ("error out"=w386:errorcluster)  [unwired: 5 in]
        n219 = call "Check Idle (non scan).vi"("error in (no error)"=w380, "Controller #"=w378, "Port In"=w379) -> ("Port Out"=w374:T6)  [unwired: 7 in, 1 out]
        n220 = call "Check Idle (non scan).vi"("error in (no error)"=w381, "Controller #"=w377, "Port In"=w379) -> ("Port Out"=w375:T6)  [unwired: 7 in, 1 out]
        n221 = call "Check Idle (non scan).vi"("error in (no error)"=w386, "Controller #"=w385, "Port In"=w379) -> ("Port Out"=w376:T6)  [unwired: 7 in, 1 out]
        n222 = flat-sequence {
          tunnel: w376 -> [w390]
          tunnel: w375 -> [_]
          tunnel: w374 -> [_]
          tunnel: [w390] -> w373
          frame #0 {
          }
        }
      }
      frame "Motor 1 Positive Relative" {
        n223 = disable-structure shown="Enabled" {
          disable-tunnel: [w402 w408] -> w395
          disable-tunnel: [w401 w407] -> w394
          disable-tunnel: w393 -> [w400 w406]
          disable-tunnel: w392 -> [w399 w405]
          frame Disabled {
            w401 = "1" ("Controller #")
            n224 = call "Move rel mMc.vi"("position incr"=w399, "Port"=w400, "rev dir?"=FALSE, "Controller #"=w401) -> ("error out"=w402:errorcluster)  [unwired: 5 in]
          }
          frame Enabled {
            w407 = "1" ("Controller #")
            n225 = call "Move rel mMc Edited.vi"("Controller #"=w407, "rev dir?"=FALSE, "Port In"=w406, "pos incr"=w405) -> ("error out"=w408:errorcluster)  [unwired: 6 in, 1 out]
          }
        }
        n226 = call "Check Idle.vi"("error in (no error)"=w395, "Controller #"=w394, "Port In"=w393) -> ("Port Out"=w391:T6)  [unwired: 7 in, 1 out]
      }
      frame "Motor 2 Positive Relative" {
        w412 = "2" ("Controller #")
        n227 = call "Move rel mMc Edited.vi"("Controller #"=w412, "rev dir?"=FALSE, "Port In"=w411, "pos incr"=w410) -> ("error out"=w413:errorcluster)  [unwired: 6 in, 1 out]
        n228 = call "Check Idle.vi"("error in (no error)"=w413, "Controller #"=w412, "Port In"=w411) -> ("Port Out"=w409:T6)  [unwired: 7 in, 1 out]
      }
      frame "Motor 3 Positive Relative" {
        w421 = "3" ("Controller #")
        n229 = call "Move rel mMc Edited.vi"("Controller #"=w421, "rev dir?"=FALSE, "Port In"=w420, "pos incr"=w419) -> ("error out"=w422:errorcluster)  [unwired: 6 in, 1 out]
        n230 = call "Check Idle.vi"("error in (no error)"=w422, "Controller #"=w421, "Port In"=w420) -> ("Port Out"=w418:T6)  [unwired: 7 in, 1 out]
      }
      frame "Motor 1 Negative Relative" {
        w430 = "1" ("Controller #")
        n231 = call "Move rel mMc Edited.vi"("Controller #"=w430, "rev dir?"=TRUE, "Port In"=w429, "pos incr"=w428) -> ("error out"=w431:errorcluster)  [unwired: 6 in, 1 out]
        n232 = call "Check Idle.vi"("error in (no error)"=w431, "Controller #"=w430, "Port In"=w429) -> ("Port Out"=w427:T6)  [unwired: 7 in, 1 out]
      }
      frame "Motor 2 Negative Relative" {
        w439 = "2" ("Controller #")
        n233 = call "Move rel mMc Edited.vi"("Controller #"=w439, "rev dir?"=TRUE, "Port In"=w438, "pos incr"=w437) -> ("error out"=w440:errorcluster)  [unwired: 6 in, 1 out]
        n234 = call "Check Idle.vi"("error in (no error)"=w440, "Controller #"=w439, "Port In"=w438) -> ("Port Out"=w436:T6)  [unwired: 7 in, 1 out]
      }
      frame "Motor 3 Negative Relative" {
        w448 = "3" ("Controller #")
        n235 = call "Move rel mMc Edited.vi"("Controller #"=w448, "rev dir?"=TRUE, "Port In"=w447, "pos incr"=w446) -> ("error out"=w449:errorcluster)  [unwired: 6 in, 1 out]
        n236 = call "Check Idle.vi"("error in (no error)"=w449, "Controller #"=w448, "Port In"=w447) -> ("Port Out"=w445:T6)  [unwired: 7 in, 1 out]
      }
      frame "Update Limits" {
        n237 = call "Travel limit negative mMc.vi"("limit in"="NL 1", "Port"=w462, "set/get"=TRUE, "Controller #"="1") -> ("error out"=w468:errorcluster)  [unwired: 4 in, 1 out]
        n238 = call "Travel limit negative mMc.vi"("limit in"="NL 2", "Port"=w462, "error in (no error)"=w468, "set/get"=TRUE, "Controller #"="2") -> ("error out"=w467:errorcluster)  [unwired: 3 in, 1 out]
        n239 = call "Travel limit negative mMc.vi"("limit in"="NL 3", "Port"=w462, "error in (no error)"=w467, "set/get"=TRUE, "Controller #"="3") -> ("error out"=w466:errorcluster)  [unwired: 3 in, 1 out]
        n240 = call "Travel limit positive mMc.vi"("limit in"="PL 1", "Port"=w462, "error in (no error)"=w466, "set/get"=TRUE, "Controller #"="1") -> ("error out"=w465:errorcluster)  [unwired: 3 in, 1 out]
        n241 = call "Travel limit positive mMc.vi"("limit in"="PL 2", "Port"=w462, "error in (no error)"=w465, "set/get"=TRUE, "Controller #"="2") -> ("error out"=w464:errorcluster)  [unwired: 3 in, 1 out]
        n242 = call "Travel limit positive mMc.vi"("limit in"="PL 3", "Port"=w462, "error in (no error)"=w464, "set/get"=TRUE, "Controller #"="3") -> ()  [unwired: 3 in, 2 out]
      }
      frame "Initialize Graph" {
        n243 = property on="Graph" class="IntGraph (strict)"("YScale.Multiplier"=w495) -> ()  [unwired: 2 in, 2 out]
        n244 = property on="Graph" class="IntGraph (strict)"("XScale.Multiplier"=w496) -> ()  [unwired: 2 in, 2 out]
        n245 = case shown="\"1\", Default" w494 {
          tunnel: [w515 w517 w519] -> w491
          frame "1", Default {
            n246 = local read "Scan Origin"() -> (w516:T1)
            n247 = Unbundle By Name(w516) -> ("Cnt pos 1"=w515:dbl)  [unwired: 2 out]
          }
          frame "2" {
            n248 = local read "Scan Origin"() -> (w518:T1)
            n249 = Unbundle By Name(w518) -> ("Cnt pos 2"=w517:dbl)  [unwired: 2 out]
          }
          frame "3" {
            n250 = local read "Scan Origin"() -> (w520:T1)
            n251 = Unbundle By Name(w520) -> ("Cnt pos 3"=w519:dbl)  [unwired: 2 out]
          }
        }
        n252 = case shown="False" "T=SP \nf=CP" {
          tunnel: w491 -> [w509 w514]
          tunnel: [w512 w514] -> w490
          tunnel: w493 -> [w510 _]
          frame False {
            n253 = Divide(x=w510, y=2.0) -> (x/y=w511:dbl)
            n254 = Subtract(x=w509, y=w511) -> (x-y=w512:dbl)
          }
          frame True {
          }
        }
        n255 = property on="Graph" class="IntGraph (strict)"("XScale.Offset"=w490) -> ()  [unwired: 2 in, 2 out]
        n256 = case shown="\"2\", Default" w486 {
          tunnel: [w504 w505 w507] -> w489
          frame "1" {
            n257 = local read "Scan Origin"() -> (w503:T1)
            n258 = Unbundle By Name(w503) -> ("Cnt pos 1"=w504:dbl)  [unwired: 2 out]
          }
          frame "2", Default {
            n259 = local read "Scan Origin"() -> (w506:T1)
            n260 = Unbundle By Name(w506) -> ("Cnt pos 2"=w505:dbl)  [unwired: 2 out]
          }
          frame "3" {
            n261 = local read "Scan Origin"() -> (w508:T1)
            n262 = Unbundle By Name(w508) -> ("Cnt pos 3"=w507:dbl)  [unwired: 2 out]
          }
        }
        n263 = local read "T=SP \nf=CP"() -> (w487:bool)
        n264 = case shown="False" w487 {
          tunnel: w489 -> [w497 w502]
          tunnel: [w500 w502] -> w488
          tunnel: w485 -> [w498 _]
          frame False {
            n265 = Divide(x=w498, y=2.0) -> (x/y=w499:dbl)
            n266 = Subtract(x=w497, y=w499) -> (x-y=w500:dbl)
          }
          frame True {
          }
        }
        n267 = local read "Scan Type"() -> (w481:string)
        n268 = property on="Graph" class="IntGraph (strict)"("YScale.Offset"=w488) -> ()  [unwired: 2 in, 2 out]
      }
      frame "Start Point Serpent Scan" {
        n269 = Divide(x=w547, y=w546) -> (x/y=w548:dbl)
        n270 = Divide(x=w534, y=w531) -> (x/y=w549:dbl)
        n271 = Round Toward +Infinity(x=w548) -> (ceil(x): smallest int >= x=w523:dbl)
        n272 = Round Toward +Infinity(x=w549) -> (ceil(x): smallest int >= x=w526:dbl)
        n273 = call "Initialize DAQ Assistant.vi"("minimum value"=w521, "maximum value"=w522, "rate"=w540, "number of samples"=w537, "physical channels"=w539) -> ("task out"=w541:refnum<k21>)  [unwired: 5 in, 1 out]
        n274 = Divide(x=w532, y=w531) -> (x/y=w530:dbl)
        n275 = Multiply(x=w523, y=w530) -> (x*y=w529:dbl)
        n276 = Increment(x=w523) -> (x+1=w524:dbl)
        n277 = Round Toward +Infinity(x=w529) -> (ceil(x): smallest int >= x=w527:dbl)
        n278 = Add(x=w526, y=w527) -> (x+y=w528:dbl)
        n279 = Increment(x=w528) -> (x+1=w545:dbl)
        n280 = Initialize Array(-inf, w545, w524) -> (w544:dbl[][])
        n281 = while {
          tunnel: w538 -> [w567]
          tunnel: w550 -> [w594]
          tunnel: w542 -> [w589]
          tunnel: w546 -> [w597]
          tunnel: w547 -> [w600]
          tunnel: w531 -> [w599]
          tunnel: w534 -> [w598]
          shift-right: [w558] -> _
          shift-left: w544 -> [w593]
          tunnel: w542 -> [w587]
          tunnel: w541 -> [w584]
          tunnel: [w582] -> w536
          tunnel: w537 -> [w581]
          tunnel: w537 -> [w580]
          tunnel: w532 -> [w569]
          tunnel: w535 -> [w570]
          tunnel: w526 -> [w564]
          tunnel: w525 -> [w565]
          tunnel: w523 -> [w555]
          i -> [w554]
          stop <- w608 stop-if-true
          n282 = Tick Count (ms)() -> (millisecond timer value=w553:u32)
          n283 = Quotient & Remainder(x=w554, y=2) -> (x-y*floor(x/y)=w605:i32)  [unwired: 1 out]
          n284 = Equal?(x=w605, y=1) -> (x = y?=w606:bool)
          n285 = Select(t=TRUE, s=w606, f=FALSE) -> (s? t:f=w586:bool)
          n286 = while {
            tunnel: w567 -> [w673]
            tunnel: w589 -> [w672]
            tunnel: w586 -> [w662]
            tunnel: w599 -> [w676]
            tunnel: w598 -> [w678]
            tunnel: [w658] -> w601
            shift-right: [w671] -> w591
            shift-left: w593 -> [w670]
            tunnel: w554 -> [w669]
            tunnel: [w666] -> w590
            tunnel: w586 -> [w665]
            tunnel: [w665] -> w585
            tunnel: w584 -> [w661]
            tunnel: [w660] -> w583
            tunnel: w581 -> [w652]
            tunnel: w565 -> [w650]
            tunnel: w564 -> [w649]
            tunnel: [w650] -> w562
            tunnel: [w649] -> w561
            i -> [w668]
            stop <- w680 stop-if-true
            n287 = flat-sequence {
              tunnel: w676 -> [w689]
              tunnel: [w688] -> w675
              tunnel: w664 -> [w687]
              tunnel: [w687] -> w663
              frame #0 {
                n288 = local read "Abort Scan"() -> (w691:bool)
                n289 = Select(t=0.0, s=w691, f=w689) -> (s? t:f=w688:dbl)
              }
            }
            n290 = call "Move rel mMc Edited.vi"("Controller #"=w673, "rev dir?"=w662, "Port In"=w672, "error in (no error)"=w663, "pos incr"=w675) -> ("error out"=w656:errorcluster, "Port Out"=w651:T5)  [unwired: 5 in]
            n291 = flat-sequence {
              tunnel: w656 -> [w681]
              tunnel: [w681] -> w655
              frame #0 {
              }
            }
            n292 = Increment(x=w668) -> (x+1=w667:i32)
            n293 = flat-sequence {
              tunnel: [w700] -> w671
              tunnel: w670 -> [w707]
              tunnel: w669 -> [w705]
              tunnel: w668 -> [w706]
              tunnel: w665 -> [w704]
              tunnel: [w703] -> w664
              tunnel: w661 -> [w702]
              tunnel: [w701] -> w660
              tunnel: w652 -> [w699]
              tunnel: w650 -> [w697]
              tunnel: w649 -> [w696]
              frame #0 {
                n294 = call "Measure and Update Array.vi"("Array In"=w707, "number of samples per channel"=w699, "task/channels in"=w702, "Row"=w706, "Column"=w705, "Invert?"=w704, "Offset"=w697, "Total Steps in Fast"=w696) -> ("Array Out"=w700:dbl[][], "task out"=w701:refnum<k21>, "Measurement"=→"Measured":dbl, "error out"=w703:errorcluster)  [unwired: 4 in]
                "Graph" <- w700
              }
            }
            n295 = call "Check Idle.vi"("error in (no error)"=w655, "Controller #"=w673, "Port In"=w651) -> ("error out (no error)"=w674:errorcluster)  [unwired: 7 in, 1 out]
            n296 = Multiply(x=w676, y=w667) -> (x*y=w677:dbl)
            n297 = Tick Count (ms)() -> (millisecond timer value=w653:u32)
            n298 = Greater Or Equal?(x=w677, y=w678) -> (x >= y?=w679:bool)
            n299 = flat-sequence {
              tunnel: [w684] -> w657
              tunnel: w654 -> [w683]
              tunnel: w653 -> [w682]
              frame #0 {
                n300 = Subtract(x=w683, y=w682) -> (x-y=w684:u32)
              }
            }
            n301 = flat-sequence {
              tunnel: [w695] -> w680
              tunnel: w679 -> [w694]
              tunnel: w674 -> [w693]
              tunnel: [w693] -> w659
              frame #0 {
                n302 = local read "Abort Scan"() -> (w692:bool)
                n303 = Or(x=w694, y=w692) -> (x .or. y?=w695:bool)
              }
            }
            n304 = Increment(x=w668) -> (x+1=w666:i32)
            n305 = flat-sequence {
              tunnel: w659 -> [w686]
              tunnel: [w686] -> w658
              tunnel: [w685] -> w654
              frame #0 {
                n306 = Tick Count (ms)() -> (millisecond timer value=w685:u32)
              }
            }
            "Time per Pixel" <- w657
          }
          n307 = Multiply(x=w597, y=w554) -> (x*y=w607:dbl)
          n308 = Greater Or Equal?(x=w607, y=w600) -> (x >= y?=w563:bool)
          n309 = flat-sequence {
            tunnel: w601 -> [w638]
            tunnel: [w637] -> w592
            tunnel: [w640] -> w558
            tunnel: w591 -> [w643]
            tunnel: w590 -> [w642]
            tunnel: w554 -> [w641]
            tunnel: w585 -> [w633]
            tunnel: w583 -> [w639]
            tunnel: [w636] -> w582
            tunnel: w580 -> [w635]
            tunnel: w562 -> [w634]
            tunnel: w561 -> [w632]
            frame #0 {
              n310 = call "Measure and Update Array.vi"("Array In"=w643, "number of samples per channel"=w635, "task/channels in"=w639, "Row"=w642, "Column"=w641, "error in"=w638, "Invert?"=w633, "Offset"=w634, "Total Steps in Fast"=w632) -> ("Array Out"=w640:dbl[][], "task out"=w636:refnum<k21>, "error out"=w637:errorcluster)  [unwired: 3 in, 1 out]
              n311 = local write "Graph"(w640) -> ()
            }
          }
          n312 = flat-sequence {
            tunnel: w597 -> [w629]
            tunnel: [w628] -> w588
            tunnel: [w627] -> w596
            tunnel: w592 -> [w627]
            frame #0 {
              n313 = local read "Abort Scan"() -> (w631:bool)
              n314 = Select(t=0.0, s=w631, f=w629) -> (s? t:f=w628:dbl)
            }
          }
          n315 = flat-sequence {
            tunnel: [w648] -> w608
            tunnel: w563 -> [w647]
            tunnel: w566 -> [w646]
            tunnel: [w646] -> _
            tunnel: [w644] -> w560
            frame #0 {
              n316 = local read "Abort Scan"() -> (w645:bool)
              n317 = Or(x=w647, y=w645) -> (x .or. y?=w648:bool)
              n318 = Tick Count (ms)() -> (millisecond timer value=w644:u32)
            }
          }
          n319 = case shown="False" w563 {
            tunnel: w596 -> [w624 w626]
            tunnel: w594 -> [w620 _]
            tunnel: w588 -> [w622 _]
            tunnel: w587 -> [w621 w625]
            tunnel: [w619 w625] -> w571
            tunnel: [w618 w626] -> w568
            frame False {
              n320 = call "Move rel mMc Edited.vi"("Controller #"=w620, "Port In"=w621, "error in (no error)"=w624, "pos incr"=w622) -> ("error out"=w623:errorcluster, "Port Out"=w617:T5)  [unwired: 6 in]
              n321 = call "Check Idle.vi"("error in (no error)"=w623, "Controller #"=w620, "Port In"=w617) -> ("error out (no error)"=w618:errorcluster, "Port Out"=w619:T6)  [unwired: 7 in]
            }
            frame True {
            }
          }
          n322 = Subtract(x=w560, y=w553) -> (x-y=w559:u32)
          n323 = property on="Graph" class="IntGraph (strict)"() -> ("XScale.Multiplier"=w576:dbl)  [unwired: 2 in, 2 out]
          n324 = property on="Graph" class="IntGraph (strict)"() -> ("YScale.Multiplier"=w578:dbl)  [unwired: 2 in, 2 out]
          n325 = property on="Graph" class="IntGraph (strict)"() -> ("XScale.Offset"=w577:dbl)  [unwired: 2 in, 2 out]
          n326 = property on="Graph" class="IntGraph (strict)"() -> ("YScale.Offset"=w579:dbl)  [unwired: 2 in, 2 out]
          n327 = call "Time Left.vi"("Time Elapsed\nper slow"=w559, "Current slow pos"=w554, "Slow array size"=w555) -> ("Estimated Time \nLeft"=→"Estimated\nTime Left":dbl, "Percent Complete"=→"Percent Complete":dbl)  [unwired: 7 in]
          n328 = flat-sequence {
            tunnel: w571 -> [w616]
            tunnel: w570 -> [w615]
            tunnel: w569 -> [w614]
            tunnel: w568 -> [w613]
            tunnel: w567 -> [w611]
            tunnel: [w609] -> w566
            frame #0 {
              n329 = call "Move rel mMc Edited.vi"("Controller #"=w611, "rev dir?"=w615, "Port In"=w616, "error in (no error)"=w613, "pos incr"=w614) -> ("error out"=w610:errorcluster, "Port Out"=w612:T5)  [unwired: 5 in]
              n330 = call "Check Idle.vi"("error in (no error)"=w610, "Controller #"=w611, "Port In"=w612) -> ("error out (no error)"=w609:errorcluster)  [unwired: 7 in, 1 out]
            }
          }
          n331 = call "Max and Min Location.vi"("Array"=w558, "x multiplier"=w576, "x offset"=w577, "y multiplier"=w578, "y offset"=w579) -> ("max value"=→"Max Value":dbl, "Fast Axis Pos (Max)"=→"Fast Axis Pos\n(Max)":dbl, "Slow Axis Pos (Max)"=→"Slow Axis Pos\n(Max)":dbl, "min value"=→"Min Value":dbl)  [unwired: 7 in]
        }
        n332 = call <vilib>:"DAQmx Clear Task.vi"("task in"=w536) -> ()  [unwired: 14 in, 1 out]
      }
      frame "Center Serpent Scan" {
        n333 = Divide(x=w738, y=w748) -> (x/y=w749:dbl)
        n334 = Divide(x=w719, y=w717) -> (x/y=w750:dbl)
        n335 = Round Toward +Infinity(x=w749) -> (ceil(x): smallest int >= x=w710:dbl)
        n336 = Round Toward +Infinity(x=w750) -> (ceil(x): smallest int >= x=w712:dbl)
        n337 = Divide(x=w738, y=2.0) -> (x/y=w737:dbl)
        n338 = Divide(x=w719, y=2.0) -> (x/y=w734:dbl)
        n339 = Divide(x=w718, y=w717) -> (x/y=w716:dbl)
        n340 = call "Initialize DAQ Assistant.vi"("minimum value"=w708, "maximum value"=w709, "rate"=w742, "number of samples"=w740, "physical channels"=w741) -> ("task out"=w743:refnum<k21>)  [unwired: 5 in, 1 out]
        n341 = call "Move rel mMc Edited.vi"("Controller #"=w726, "rev dir?"=TRUE, "Port In"=w732, "pos incr"=w734) -> ("error out"=w727:errorcluster, "Port Out"=w728:T5)  [unwired: 6 in]
        n342 = Multiply(x=w710, y=w716) -> (x*y=w715:dbl)
        n343 = call "Move rel mMc Edited.vi"("Controller #"=w730, "rev dir?"=TRUE, "Port In"=w732, "pos incr"=w737) -> ("error out"=w729:errorcluster, "Port Out"=w731:T5)  [unwired: 6 in]
        n344 = Round Toward +Infinity(x=w715) -> (ceil(x): smallest int >= x=w713:dbl)
        n345 = Add(x=w712, y=w713) -> (x+y=w714:dbl)
        n346 = Increment(x=w710) -> (x+1=w747:dbl)
        n347 = Increment(x=w714) -> (x+1=w746:dbl)
        n348 = call "Check Idle (non scan).vi"("error in (no error)"=w727, "Controller #"=w726, "Port In"=w728) -> ("Port Out"=w725:T6)  [unwired: 7 in, 1 out]
        n349 = call "Check Idle (non scan).vi"("error in (no error)"=w729, "Controller #"=w730, "Port In"=w731) -> ("Port Out"=w724:T6)  [unwired: 7 in, 1 out]
        n350 = Initialize Array(-inf, w746, w747) -> (w745:dbl[][])
        n351 = flat-sequence {
          tunnel: w725 -> [w753]
          tunnel: w724 -> [_]
          tunnel: [w753] -> w723
          frame #0 {
          }
        }
        n352 = while {
          tunnel: w726 -> [w768]
          tunnel: w730 -> [w795]
          tunnel: w723 -> [w790]
          tunnel: w748 -> [w798]
          tunnel: w738 -> [w801]
          tunnel: w717 -> [w800]
          tunnel: w719 -> [w799]
          shift-right: [w761] -> _
          shift-left: w745 -> [w794]
          tunnel: w732 -> [w788]
          tunnel: w743 -> [w785]
          tunnel: w740 -> [w782]
          tunnel: w740 -> [w781]
          tunnel: [w783] -> w722
          tunnel: w718 -> [w769]
          tunnel: w721 -> [w770]
          tunnel: w712 -> [w766]
          tunnel: w711 -> [w767]
          tunnel: w710 -> [w757]
          i -> [w756]
          stop <- w809 stop-if-true
          n353 = Quotient & Remainder(x=w756, y=2) -> (x-y*floor(x/y)=w806:i32)  [unwired: 1 out]
          n354 = Equal?(x=w806, y=1) -> (x = y?=w807:bool)
          n355 = Select(t=TRUE, s=w807, f=FALSE) -> (s? t:f=w787:bool)
          n356 = while {
            tunnel: w768 -> [w874]
            tunnel: w790 -> [w873]
            tunnel: w787 -> [w863]
            tunnel: w800 -> [w877]
            tunnel: w799 -> [w879]
            tunnel: [w859] -> w802
            shift-right: [w872] -> w792
            shift-left: w794 -> [w871]
            tunnel: w756 -> [w870]
            tunnel: [w867] -> w791
            tunnel: w787 -> [w866]
            tunnel: [w866] -> w786
            tunnel: w785 -> [w862]
            tunnel: [w861] -> w784
            tunnel: w782 -> [w854]
            tunnel: w767 -> [w851]
            tunnel: w766 -> [w850]
            tunnel: [w851] -> w764
            tunnel: [w850] -> w762
            i -> [w869]
            stop <- w881 stop-if-true
            n357 = flat-sequence {
              tunnel: w877 -> [w890]
              tunnel: [w889] -> w876
              tunnel: w865 -> [w888]
              tunnel: [w888] -> w864
              frame #0 {
                n358 = local read "Abort Scan"() -> (w892:bool)
                n359 = Select(t=0.0, s=w892, f=w890) -> (s? t:f=w889:dbl)
              }
            }
            n360 = call "Move rel mMc Edited.vi"("Controller #"=w874, "rev dir?"=w863, "Port In"=w873, "error in (no error)"=w864, "pos incr"=w876) -> ("error out"=w858:errorcluster, "Port Out"=w852:T5)  [unwired: 5 in]
            n361 = flat-sequence {
              tunnel: w858 -> [w882]
              tunnel: [w882] -> w857
              frame #0 {
              }
            }
            n362 = Increment(x=w869) -> (x+1=w868:i32)
            n363 = flat-sequence {
              tunnel: [w900] -> w872
              tunnel: w871 -> [w908]
              tunnel: w870 -> [w906]
              tunnel: w869 -> [w907]
              tunnel: w866 -> [w905]
              tunnel: [w904] -> w865
              tunnel: w862 -> [w903]
              tunnel: [w902] -> w861
              tunnel: w854 -> [w901]
              tunnel: w851 -> [w898]
              tunnel: w850 -> [w897]
              frame #0 {
                n364 = call "Measure and Update Array.vi"("Array In"=w908, "number of samples per channel"=w901, "task/channels in"=w903, "Row"=w907, "Column"=w906, "Invert?"=w905, "Offset"=w898, "Total Steps in Fast"=w897) -> ("Array Out"=w900:dbl[][], "task out"=w902:refnum<k21>, "Measurement"=w899:dbl, "error out"=w904:errorcluster)  [unwired: 4 in]
                n365 = local write "Graph"(w900) -> ()
                n366 = local write "Measured"(w899) -> ()
              }
            }
            n367 = call "Check Idle.vi"("error in (no error)"=w857, "Controller #"=w874, "Port In"=w852) -> ("error out (no error)"=w875:errorcluster)  [unwired: 7 in, 1 out]
            n368 = Multiply(x=w877, y=w868) -> (x*y=w878:dbl)
            n369 = Tick Count (ms)() -> (millisecond timer value=w855:u32)
            n370 = Greater Or Equal?(x=w878, y=w879) -> (x >= y?=w880:bool)
            n371 = flat-sequence {
              tunnel: [w896] -> w881
              tunnel: w880 -> [w895]
              tunnel: w875 -> [w894]
              tunnel: [w894] -> w860
              frame #0 {
                n372 = local read "Abort Scan"() -> (w893:bool)
                n373 = Or(x=w895, y=w893) -> (x .or. y?=w896:bool)
              }
            }
            n374 = flat-sequence {
              tunnel: [w885] -> w853
              tunnel: w856 -> [w884]
              tunnel: w855 -> [w883]
              frame #0 {
                n375 = Subtract(x=w884, y=w883) -> (x-y=w885:u32)
              }
            }
            n376 = Increment(x=w869) -> (x+1=w867:i32)
            n377 = flat-sequence {
              tunnel: w860 -> [w887]
              tunnel: [w887] -> w859
              tunnel: [w886] -> w856
              frame #0 {
                n378 = Tick Count (ms)() -> (millisecond timer value=w886:u32)
              }
            }
            n379 = local write "Time per Pixel"(w853) -> ()
          }
          n380 = Multiply(x=w798, y=w756) -> (x*y=w808:dbl)
          n381 = Greater Or Equal?(x=w808, y=w801) -> (x >= y?=w765:bool)
          n382 = Tick Count (ms)() -> (millisecond timer value=w759:u32)
          n383 = flat-sequence {
            tunnel: w802 -> [w838]
            tunnel: [w837] -> w793
            tunnel: [w840] -> w761
            tunnel: w792 -> [w844]
            tunnel: w791 -> [w843]
            tunnel: w756 -> [w842]
            tunnel: w786 -> [w841]
            tunnel: w784 -> [w839]
            tunnel: [w836] -> w783
            tunnel: w781 -> [w835]
            tunnel: w764 -> [w834]
            tunnel: w762 -> [w833]
            frame #0 {
              n384 = call "Measure and Update Array.vi"("Array In"=w844, "number of samples per channel"=w835, "task/channels in"=w839, "Row"=w843, "Column"=w842, "error in"=w838, "Invert?"=w841, "Offset"=w834, "Total Steps in Fast"=w833) -> ("Array Out"=w840:dbl[][], "task out"=w836:refnum<k21>, "error out"=w837:errorcluster)  [unwired: 3 in, 1 out]
              n385 = local write "Graph"(w840) -> ()
            }
          }
          n386 = flat-sequence {
            tunnel: w798 -> [w830]
            tunnel: [w829] -> w789
            tunnel: [w828] -> w797
            tunnel: w793 -> [w828]
            frame #0 {
              n387 = local read "Abort Scan"() -> (w832:bool)
              n388 = Select(t=0.0, s=w832, f=w830) -> (s? t:f=w829:dbl)
            }
          }
          n389 = flat-sequence {
            tunnel: [w849] -> w809
            tunnel: w765 -> [w848]
            tunnel: w763 -> [w846]
            tunnel: [w846] -> _
            tunnel: [w845] -> w760
            frame #0 {
              n390 = local read "Abort Scan"() -> (w847:bool)
              n391 = Tick Count (ms)() -> (millisecond timer value=w845:u32)
              n392 = Or(x=w848, y=w847) -> (x .or. y?=w849:bool)
            }
          }
          n393 = Subtract(x=w760, y=w759) -> (x-y=w758:u32)
          n394 = case shown="False" w765 {
            tunnel: w797 -> [w825 w826]
            tunnel: w795 -> [w821 _]
            tunnel: w789 -> [w823 _]
            tunnel: w788 -> [w822 w827]
            tunnel: [w820 w826] -> w772
            tunnel: [w819 w827] -> w771
            frame False {
              n395 = call "Move rel mMc Edited.vi"("Controller #"=w821, "Port In"=w822, "error in (no error)"=w825, "pos incr"=w823) -> ("error out"=w824:errorcluster, "Port Out"=w818:T5)  [unwired: 6 in]
              n396 = call "Check Idle.vi"("error in (no error)"=w824, "Controller #"=w821, "Port In"=w818) -> ("error out (no error)"=w820:errorcluster, "Port Out"=w819:T6)  [unwired: 7 in]
            }
            frame True {
            }
          }
          n397 = call "Time Left.vi"("Time Elapsed\nper slow"=w758, "Current slow pos"=w756, "Slow array size"=w757) -> ("Estimated Time \nLeft"=w754:dbl, "Percent Complete"=w755:dbl)  [unwired: 7 in]
          n398 = property on="Graph" class="IntGraph (strict)"() -> ("XScale.Multiplier"=w773:dbl)  [unwired: 2 in, 2 out]
          n399 = property on="Graph" class="IntGraph (strict)"() -> ("YScale.Multiplier"=w775:dbl)  [unwired: 2 in, 2 out]
          n400 = property on="Graph" class="IntGraph (strict)"() -> ("XScale.Offset"=w774:dbl)  [unwired: 2 in, 2 out]
          n401 = property on="Graph" class="IntGraph (strict)"() -> ("YScale.Offset"=w776:dbl)  [unwired: 2 in, 2 out]
          n402 = local write "Estimated\nTime Left"(w754) -> ()
          n403 = local write "Percent Complete"(w755) -> ()
          n404 = flat-sequence {
            tunnel: w771 -> [w817]
            tunnel: w770 -> [w816]
            tunnel: w769 -> [w815]
            tunnel: w772 -> [w814]
            tunnel: w768 -> [w812]
            tunnel: [w810] -> w763
            frame #0 {
              n405 = call "Move rel mMc Edited.vi"("Controller #"=w812, "rev dir?"=w816, "Port In"=w817, "error in (no error)"=w814, "pos incr"=w815) -> ("error out"=w811:errorcluster, "Port Out"=w813:T5)  [unwired: 5 in]
              n406 = call "Check Idle.vi"("error in (no error)"=w811, "Controller #"=w812, "Port In"=w813) -> ("error out (no error)"=w810:errorcluster)  [unwired: 7 in, 1 out]
            }
          }
          n407 = call "Max and Min Location.vi"("Array"=w761, "x multiplier"=w773, "x offset"=w774, "y multiplier"=w775, "y offset"=w776) -> ("max value"=w777:dbl, "Fast Axis Pos (Max)"=w778:dbl, "Slow Axis Pos (Max)"=w779:dbl, "min value"=w780:dbl)  [unwired: 7 in]
          n408 = local write "Slow Axis Pos\n(Max)"(w779) -> ()
          n409 = local write "Fast Axis Pos\n(Max)"(w778) -> ()
          n410 = local write "Min Value"(w780) -> ()
          n411 = local write "Max Value"(w777) -> ()
        }
        n412 = call <vilib>:"DAQmx Clear Task.vi"("task in"=w722) -> ()  [unwired: 14 in, 1 out]
      }
      frame "Start Point Typewriter Scan" {
        n413 = Divide(x=w924, y=w935) -> (x/y=w937:dbl)
        n414 = Divide(x=w921, y=w920) -> (x/y=w936:dbl)
        n415 = Round Toward +Infinity(x=w937) -> (ceil(x): smallest int >= x=w912:dbl)
        n416 = Round Toward +Infinity(x=w936) -> (ceil(x): smallest int >= x=w914:dbl)
        n417 = Divide(x=w919, y=w920) -> (x/y=w918:dbl)
        n418 = call "Initialize DAQ Assistant.vi"("minimum value"=w909, "maximum value"=w910, "rate"=w928, "number of samples"=w925, "physical channels"=w926) -> ("task out"=w927:refnum<k21>)  [unwired: 5 in, 1 out]
        n419 = Multiply(x=w912, y=w918) -> (x*y=w917:dbl)
        n420 = Round Toward +Infinity(x=w917) -> (ceil(x): smallest int >= x=w916:dbl)
        n421 = Add(x=w914, y=w916) -> (x+y=w915:dbl)
        n422 = Increment(x=w915) -> (x+1=w933:dbl)
        n423 = Increment(x=w912) -> (x+1=w932:dbl)
        n424 = Initialize Array(-inf, w933, w932) -> (w934:dbl[][])
        n425 = while {
          tunnel: w938 -> [w995]
          tunnel: w931 -> [w973]
          tunnel: w929 -> [w985]
          tunnel: w935 -> [w984]
          tunnel: w924 -> [w993]
          tunnel: w920 -> [w992]
          tunnel: w921 -> [w991]
          tunnel: w929 -> [w974]
          tunnel: w938 -> [w953]
          shift-right: [w959] -> _
          shift-left: w934 -> [w980]
          tunnel: [w971] -> w911
          tunnel: w927 -> [w970]
          tunnel: w925 -> [w969]
          tunnel: w919 -> [w957]
          tunnel: w922 -> [w956]
          tunnel: w914 -> [w950]
          tunnel: w913 -> [w951]
          tunnel: w912 -> [w944]
          i -> [w943]
          stop <- w996 stop-if-true
          n426 = while {
            tunnel: w995 -> [w1060]
            tunnel: w985 -> [w1053]
            tunnel: w992 -> [w1063]
            tunnel: w991 -> [w1066]
            tunnel: [w1055] -> w982
            tunnel: [w1065] -> w988
            tunnel: w943 -> [w1058]
            shift-right: [w1057] -> w979
            shift-left: w980 -> [w1059]
            tunnel: [w1054] -> w978
            tunnel: [w1049] -> w972
            tunnel: w970 -> [w1048]
            tunnel: w969 -> [w1047]
            tunnel: [w1047] -> w968
            tunnel: w951 -> [w1042]
            tunnel: w950 -> [w1041]
            tunnel: [w1042] -> w949
            tunnel: [w1041] -> w948
            i -> [w1056]
            stop <- w1069 stop-if-true
            n427 = flat-sequence {
              tunnel: w1063 -> [w1075]
              tunnel: [w1074] -> w1064
              tunnel: w1051 -> [w1073]
              tunnel: [w1073] -> w1050
              frame #0 {
                n428 = local read "Abort Scan"() -> (w1077:bool)
                n429 = Select(t=0.0, s=w1077, f=w1075) -> (s? t:f=w1074:dbl)
              }
            }
            n430 = call "Move rel mMc Edited.vi"("Controller #"=w1060, "rev dir?"=FALSE, "Port In"=w1053, "error in (no error)"=w1050, "pos incr"=w1064) -> ("error out"=w1062:errorcluster, "Port Out"=w1043:T5)  [unwired: 5 in]
            n431 = Increment(x=w1056) -> (x+1=w1068:i32)
            n432 = flat-sequence {
              tunnel: w1059 -> [w1094]
              tunnel: w1058 -> [w1092]
              tunnel: w1056 -> [w1093]
              tunnel: [w1090] -> w1057
              tunnel: [w1087] -> w1051
              tunnel: [w1089] -> w1049
              tunnel: w1048 -> [w1088]
              tunnel: w1047 -> [w1086]
              tunnel: w1042 -> [w1084]
              tunnel: w1041 -> [w1083]
              frame #0 {
                n433 = call "Measure and Update Array.vi"("Array In"=w1094, "number of samples per channel"=w1086, "task/channels in"=w1088, "Row"=w1093, "Column"=w1092, "Invert?"=FALSE, "Offset"=w1084, "Total Steps in Fast"=w1083) -> ("Array Out"=w1090:dbl[][], "task out"=w1089:refnum<k21>, "Measurement"=w1085:dbl, "error out"=w1087:errorcluster)  [unwired: 4 in]
                n434 = local write "Measured"(w1085) -> ()
                n435 = local write "Graph"(w1090) -> ()
              }
            }
            n436 = Multiply(x=w1063, y=w1068) -> (x*y=w1065:dbl)
            n437 = call "Check Idle.vi"("error in (no error)"=w1062, "Controller #"=w1060, "Port In"=w1043) -> ("error out (no error)"=w1061:errorcluster)  [unwired: 7 in, 1 out]
            n438 = Tick Count (ms)() -> (millisecond timer value=w1046:u32)
            n439 = Greater Or Equal?(x=w1065, y=w1066) -> (x >= y?=w1067:bool)
            n440 = flat-sequence {
              tunnel: w1046 -> [w1072]
              tunnel: w1045 -> [w1071]
              tunnel: [w1070] -> w1044
              frame #0 {
                n441 = Subtract(x=w1071, y=w1072) -> (x-y=w1070:u32)
              }
            }
            n442 = flat-sequence {
              tunnel: [w1082] -> w1069
              tunnel: w1067 -> [w1081]
              tunnel: w1061 -> [w1080]
              tunnel: [w1080] -> w1055
              tunnel: [w1078] -> w1045
              frame #0 {
                n443 = local read "Abort Scan"() -> (w1079:bool)
                n444 = Tick Count (ms)() -> (millisecond timer value=w1078:u32)
                n445 = Or(x=w1081, y=w1079) -> (x .or. y?=w1082:bool)
              }
            }
            n446 = Increment(x=w1056) -> (x+1=w1054:i32)
            n447 = local write "Time per Pixel"(w1044) -> ()
          }
          n448 = Multiply(x=w984, y=w943) -> (x*y=w994:dbl)
          n449 = Greater Or Equal?(x=w994, y=w993) -> (x >= y?=w975:bool)
          n450 = Tick Count (ms)() -> (millisecond timer value=w946:u32)
          n451 = flat-sequence {
            tunnel: w988 -> [w1022]
            tunnel: [w1021] -> w987
            frame #0 {
              n452 = local read "Abort Scan"() -> (w1024:bool)
              n453 = Select(t=0.0, s=w1024, f=w1022) -> (s? t:f=w1021:dbl)
            }
          }
          n454 = flat-sequence {
            tunnel: w982 -> [w1030]
            tunnel: [w1029] -> w990
            tunnel: w979 -> [w1036]
            tunnel: w943 -> [w1034]
            tunnel: w978 -> [w1035]
            tunnel: [w1032] -> w959
            tunnel: w972 -> [w1031]
            tunnel: [w1028] -> w971
            tunnel: w968 -> [w1027]
            tunnel: w949 -> [w1026]
            tunnel: w948 -> [w1025]
            frame #0 {
              n455 = call "Measure and Update Array.vi"("Array In"=w1036, "number of samples per channel"=w1027, "task/channels in"=w1031, "Row"=w1035, "Column"=w1034, "error in"=w1030, "Invert?"=FALSE, "Offset"=w1026, "Total Steps in Fast"=w1025) -> ("Array Out"=w1032:dbl[][], "task out"=w1028:refnum<k21>, "error out"=w1029:errorcluster)  [unwired: 3 in, 1 out]
              n456 = local write "Graph"(w1032) -> ()
            }
          }
          n457 = flat-sequence {
            tunnel: w984 -> [w1018]
            tunnel: [w1017] -> w981
            tunnel: w983 -> [w1016]
            tunnel: [w1016] -> w977
            frame #0 {
              n458 = local read "Back scan delay"() -> (w1015:u32)
              n459 = local read "Abort Scan"() -> (w1020:bool)
              n460 = Wait (ms)(milliseconds to wait=w1015) -> ()  [unwired: 1 out]
              n461 = Select(t=0.0, s=w1020, f=w1018) -> (s? t:f=w1017:dbl)
            }
          }
          n462 = flat-sequence {
            tunnel: [w1040] -> w996
            tunnel: w975 -> [w1039]
            tunnel: w954 -> [_]
            tunnel: [w1037] -> w947
            frame #0 {
              n463 = Tick Count (ms)() -> (millisecond timer value=w1037:u32)
              n464 = Or(x=w1039, y="Abort Scan") -> (x .or. y?=w1040:bool)
            }
          }
          n465 = call "Move rel mMc Edited.vi"("Controller #"=w953, "rev dir?"=TRUE, "Port In"=w974, "error in (no error)"=w990, "pos incr"=w987) -> ("error out"=w986:errorcluster, "Port Out"=w952:T5)  [unwired: 5 in]
          n466 = call "Check Idle.vi"("error in (no error)"=w986, "Controller #"=w953, "Port In"=w952) -> ("error out (no error)"=w983:errorcluster, "Port Out"=w976:T6)  [unwired: 7 in]
          n467 = case shown="False" w975 {
            tunnel: [w1011 w1014] -> w955
            tunnel: w981 -> [w1010 _]
            tunnel: w977 -> [w1009 w1014]
            tunnel: w973 -> [w1008 _]
            tunnel: w976 -> [w1007 w1013]
            tunnel: [w1006 w1013] -> w958
            frame False {
              n468 = call "Move rel mMc Edited.vi"("Controller #"=w1008, "Port In"=w1007, "error in (no error)"=w1009, "pos incr"=w1010) -> ("error out"=w1012:errorcluster, "Port Out"=w1005:T5)  [unwired: 6 in]
              n469 = call "Check Idle.vi"("error in (no error)"=w1012, "Controller #"=w1008, "Port In"=w1005) -> ("error out (no error)"=w1011:errorcluster, "Port Out"=w1006:T6)  [unwired: 7 in]
            }
            frame True {
            }
          }
          n470 = property on="Graph" class="IntGraph (strict)"() -> ("XScale.Multiplier"=w967:dbl)  [unwired: 2 in, 2 out]
          n471 = property on="Graph" class="IntGraph (strict)"() -> ("XScale.Offset"=w962:dbl)  [unwired: 2 in, 2 out]
          n472 = property on="Graph" class="IntGraph (strict)"() -> ("YScale.Multiplier"=w961:dbl)  [unwired: 2 in, 2 out]
          n473 = property on="Graph" class="IntGraph (strict)"() -> ("YScale.Offset"=w960:dbl)  [unwired: 2 in, 2 out]
          n474 = Subtract(x=w947, y=w946) -> (x-y=w945:u32)
          n475 = call "Time Left.vi"("Time Elapsed\nper slow"=w945, "Current slow pos"=w943, "Slow array size"=w944) -> ("Estimated Time \nLeft"=w941:dbl, "Percent Complete"=w942:dbl)  [unwired: 7 in]
          n476 = flat-sequence {
            tunnel: w958 -> [w1004]
            tunnel: w956 -> [w1003]
            tunnel: w957 -> [w1002]
            tunnel: w955 -> [w1001]
            tunnel: w953 -> [w999]
            tunnel: [w997] -> w954
            frame #0 {
              n477 = call "Move rel mMc Edited.vi"("Controller #"=w999, "rev dir?"=w1003, "Port In"=w1004, "error in (no error)"=w1001, "pos incr"=w1002) -> ("error out"=w998:errorcluster, "Port Out"=w1000:T5)  [unwired: 5 in]
              n478 = call "Check Idle.vi"("error in (no error)"=w998, "Controller #"=w999, "Port In"=w1000) -> ("error out (no error)"=w997:errorcluster)  [unwired: 7 in, 1 out]
            }
          }
          n479 = call "Max and Min Location.vi"("Array"=w959, "x multiplier"=w967, "x offset"=w962, "y multiplier"=w961, "y offset"=w960) -> ("max value"=w964:dbl, "Fast Axis Pos (Max)"=w965:dbl, "Slow Axis Pos (Max)"=w966:dbl, "min value"=w963:dbl)  [unwired: 7 in]
          n480 = local write "Estimated\nTime Left"(w941) -> ()
          n481 = local write "Max Value"(w964) -> ()
          n482 = local write "Percent Complete"(w942) -> ()
          n483 = local write "Fast Axis Pos\n(Max)"(w965) -> ()
          n484 = local write "Slow Axis Pos\n(Max)"(w966) -> ()
          n485 = local write "Min Value"(w963) -> ()
        }
        n486 = call <vilib>:"DAQmx Clear Task.vi"("task in"=w911) -> ()  [unwired: 14 in, 1 out]
      }
      frame "Center Typewriter Scan" {
        n487 = Divide(x=w1109, y=w1100) -> (x/y=w1137:dbl)
        n488 = Divide(x=w1125, y=w1136) -> (x/y=w1138:dbl)
        n489 = Divide(x=w1125, y=2.0) -> (x/y=w1112:dbl)
        n490 = Divide(x=w1109, y=2.0) -> (x/y=w1121:dbl)
        n491 = Round Toward +Infinity(x=w1137) -> (ceil(x): smallest int >= x=w1103:dbl)
        n492 = Round Toward +Infinity(x=w1138) -> (ceil(x): smallest int >= x=w1099:dbl)
        n493 = Divide(x=w1101, y=w1100) -> (x/y=w1102:dbl)
        n494 = Multiply(x=w1099, y=w1102) -> (x*y=w1108:dbl)
        n495 = call "Move rel mMc Edited.vi"("Controller #"=w1116, "rev dir?"=TRUE, "Port In"=w1107, "pos incr"=w1121) -> ("error out"=w1118:errorcluster, "Port Out"=w1119:T5)  [unwired: 6 in]
        n496 = call "Initialize DAQ Assistant.vi"("minimum value"=w1096, "maximum value"=w1097, "rate"=w1131, "number of samples"=w1128, "physical channels"=w1129) -> ("task out"=w1130:refnum<k21>)  [unwired: 5 in, 1 out]
        n497 = call "Move rel mMc Edited.vi"("Controller #"=w1106, "rev dir?"=TRUE, "Port In"=w1107, "pos incr"=w1112) -> ("error out"=w1123:errorcluster, "Port Out"=w1124:T5)  [unwired: 6 in]
        n498 = Round Toward +Infinity(x=w1108) -> (ceil(x): smallest int >= x=w1104:dbl)
        n499 = Add(x=w1103, y=w1104) -> (x+y=w1105:dbl)
        n500 = call "Check Idle (non scan).vi"("error in (no error)"=w1118, "Controller #"=w1116, "Port In"=w1119) -> ("Port Out"=w1115:T6)  [unwired: 7 in, 1 out]
        n501 = Increment(x=w1105) -> (x+1=w1134:dbl)
        n502 = Increment(x=w1099) -> (x+1=w1133:dbl)
        n503 = call "Check Idle (non scan).vi"("error in (no error)"=w1123, "Controller #"=w1106, "Port In"=w1124) -> ("Port Out"=w1114:T6)  [unwired: 7 in, 1 out]
        n504 = Initialize Array(-inf, w1134, w1133) -> (w1135:dbl[][])
        n505 = flat-sequence {
          tunnel: w1115 -> [w1141]
          tunnel: w1114 -> [_]
          tunnel: [w1141] -> w1113
          frame #0 {
          }
        }
        n506 = while {
          tunnel: w1116 -> [w1154]
          tunnel: w1106 -> [w1177]
          tunnel: w1113 -> [w1188]
          tunnel: w1136 -> [w1187]
          tunnel: w1125 -> [w1195]
          tunnel: w1100 -> [w1194]
          tunnel: w1109 -> [w1162]
          tunnel: w1107 -> [w1178]
          shift-right: [w1161] -> _
          shift-left: w1135 -> [w1183]
          tunnel: w1130 -> [w1175]
          tunnel: w1128 -> [w1174]
          tunnel: [w1163] -> w1098
          tunnel: w1101 -> [w1157]
          tunnel: w1111 -> [w1156]
          tunnel: w1110 -> [w1153]
          tunnel: w1103 -> [w1152]
          tunnel: w1099 -> [w1144]
          tunnel: "Time To Wait" -> [w1142]
          i -> [w1143]
          stop <- w1197 stop-if-true
          n507 = while {
            tunnel: w1154 -> [w1263]
            tunnel: w1188 -> [w1256]
            tunnel: w1194 -> [w1266]
            tunnel: w1162 -> [w1269]
            tunnel: [w1258] -> w1185
            tunnel: [w1268] -> w1191
            tunnel: w1143 -> [w1261]
            shift-right: [w1260] -> w1182
            shift-left: w1183 -> [w1262]
            tunnel: [w1257] -> w1181
            tunnel: [w1252] -> w1176
            tunnel: w1175 -> [w1244]
            tunnel: w1174 -> [w1251]
            tunnel: [w1251] -> w1173
            tunnel: w1153 -> [w1246]
            tunnel: w1152 -> [w1245]
            tunnel: [w1246] -> w1151
            tunnel: [w1245] -> w1150
            tunnel: w1142 -> [w1242]
            i -> [w1259]
            stop <- w1272 stop-if-true
            n508 = flat-sequence {
              tunnel: w1266 -> [w1280]
              tunnel: [w1279] -> w1267
              tunnel: w1254 -> [w1278]
              tunnel: [w1278] -> w1253
              frame #0 {
                n509 = local read "Abort Scan"() -> (w1282:bool)
                n510 = Select(t=0.0, s=w1282, f=w1280) -> (s? t:f=w1279:dbl)
              }
            }
            n511 = flat-sequence {
              tunnel: w1244 -> [w1274]
              tunnel: [w1274] -> w1243
              tunnel: w1242 -> [w1273]
              frame #0 {
                n512 = Wait (ms)(milliseconds to wait=w1273) -> ()  [unwired: 1 out]
              }
            }
            n513 = call "Move rel mMc Edited.vi"("Controller #"=w1263, "rev dir?"=FALSE, "Port In"=w1256, "error in (no error)"=w1253, "pos incr"=w1267) -> ("error out"=w1265:errorcluster, "Port Out"=w1247:T5)  [unwired: 5 in]
            n514 = Increment(x=w1259) -> (x+1=w1271:i32)
            n515 = flat-sequence {
              tunnel: w1262 -> [w1299]
              tunnel: w1261 -> [w1297]
              tunnel: w1259 -> [w1298]
              tunnel: [w1295] -> w1260
              tunnel: [w1292] -> w1254
              tunnel: [w1294] -> w1252
              tunnel: w1243 -> [w1293]
              tunnel: w1251 -> [w1291]
              tunnel: w1246 -> [w1289]
              tunnel: w1245 -> [w1288]
              frame #0 {
                n516 = call "Measure and Update Array.vi"("Array In"=w1299, "number of samples per channel"=w1291, "task/channels in"=w1293, "Row"=w1298, "Column"=w1297, "Invert?"=FALSE, "Offset"=w1289, "Total Steps in Fast"=w1288) -> ("Array Out"=w1295:dbl[][], "task out"=w1294:refnum<k21>, "Measurement"=w1290:dbl, "error out"=w1292:errorcluster)  [unwired: 4 in]
                n517 = local write "Measured"(w1290) -> ()
                n518 = local write "Graph"(w1295) -> ()
              }
            }
            n519 = Tick Count (ms)() -> (millisecond timer value=w1250:u32)
            n520 = Multiply(x=w1266, y=w1271) -> (x*y=w1268:dbl)
            n521 = call "Check Idle.vi"("error in (no error)"=w1265, "Controller #"=w1263, "Port In"=w1247) -> ("error out (no error)"=w1264:errorcluster)  [unwired: 7 in, 1 out]
            n522 = flat-sequence {
              tunnel: w1250 -> [w1277]
              tunnel: w1249 -> [w1276]
              tunnel: [w1275] -> w1248
              frame #0 {
                n523 = Subtract(x=w1276, y=w1277) -> (x-y=w1275:u32)
              }
            }
            n524 = Greater Or Equal?(x=w1268, y=w1269) -> (x >= y?=w1270:bool)
            n525 = flat-sequence {
              tunnel: [w1287] -> w1272
              tunnel: w1270 -> [w1286]
              tunnel: w1264 -> [w1285]
              tunnel: [w1285] -> w1258
              tunnel: [w1283] -> w1249
              frame #0 {
                n526 = local read "Abort Scan"() -> (w1284:bool)
                n527 = Tick Count (ms)() -> (millisecond timer value=w1283:u32)
                n528 = Or(x=w1286, y=w1284) -> (x .or. y?=w1287:bool)
              }
            }
            n529 = Increment(x=w1259) -> (x+1=w1257:i32)
            n530 = local write "Time per Pixel"(w1248) -> ()
          }
          n531 = Multiply(x=w1187, y=w1143) -> (x*y=w1196:dbl)
          n532 = Greater Or Equal?(x=w1196, y=w1195) -> (x >= y?=w1179:bool)
          n533 = Tick Count (ms)() -> (millisecond timer value=w1148:u32)
          n534 = flat-sequence {
            tunnel: w1191 -> [w1223]
            tunnel: [w1222] -> w1190
            frame #0 {
              n535 = local read "Abort Scan"() -> (w1225:bool)
              n536 = Select(t=0.0, s=w1225, f=w1223) -> (s? t:f=w1222:dbl)
            }
          }
          n537 = flat-sequence {
            tunnel: w1185 -> [w1231]
            tunnel: [w1230] -> w1193
            tunnel: w1182 -> [w1237]
            tunnel: w1143 -> [w1235]
            tunnel: w1181 -> [w1236]
            tunnel: [w1233] -> w1161
            tunnel: w1176 -> [w1232]
            tunnel: [w1229] -> w1163
            tunnel: w1173 -> [w1228]
            tunnel: w1151 -> [w1227]
            tunnel: w1150 -> [w1226]
            frame #0 {
              n538 = call "Measure and Update Array.vi"("Array In"=w1237, "number of samples per channel"=w1228, "task/channels in"=w1232, "Row"=w1236, "Column"=w1235, "error in"=w1231, "Invert?"=FALSE, "Offset"=w1227, "Total Steps in Fast"=w1226) -> ("Array Out"=w1233:dbl[][], "task out"=w1229:refnum<k21>, "error out"=w1230:errorcluster)  [unwired: 3 in, 1 out]
              n539 = local write "Graph"(w1233) -> ()
            }
          }
          n540 = flat-sequence {
            tunnel: w1187 -> [w1219]
            tunnel: [w1218] -> w1184
            tunnel: w1186 -> [w1217]
            tunnel: [w1217] -> w1180
            frame #0 {
              n541 = local read "Abort Scan"() -> (w1221:bool)
              n542 = Wait (ms)(milliseconds to wait="Back scan delay") -> ()  [unwired: 1 out]
              n543 = Select(t=0.0, s=w1221, f=w1219) -> (s? t:f=w1218:dbl)
            }
          }
          n544 = flat-sequence {
            tunnel: [w1241] -> w1197
            tunnel: w1179 -> [w1240]
            tunnel: w1159 -> [_]
            tunnel: [w1238] -> w1149
            frame #0 {
              n545 = local read "Abort Scan"() -> (w1239:bool)
              n546 = Tick Count (ms)() -> (millisecond timer value=w1238:u32)
              n547 = Or(x=w1240, y=w1239) -> (x .or. y?=w1241:bool)
            }
          }
          n548 = call "Move rel mMc Edited.vi"("Controller #"=w1154, "rev dir?"=TRUE, "Port In"=w1178, "error in (no error)"=w1193, "pos incr"=w1190) -> ("error out"=w1189:errorcluster, "Port Out"=w1158:T5)  [unwired: 5 in]
          n549 = call "Check Idle.vi"("error in (no error)"=w1189, "Controller #"=w1154, "Port In"=w1158) -> ("error out (no error)"=w1186:errorcluster, "Port Out"=w1165:T6)  [unwired: 7 in]
          n550 = case shown="False" w1179 {
            tunnel: [w1212 w1215] -> w1160
            tunnel: w1184 -> [w1211 _]
            tunnel: w1180 -> [w1210 w1215]
            tunnel: w1177 -> [w1209 _]
            tunnel: w1165 -> [w1208 w1214]
            tunnel: [w1207 w1214] -> w1155
            frame False {
              n551 = call "Move rel mMc Edited.vi"("Controller #"=w1209, "Port In"=w1208, "error in (no error)"=w1210, "pos incr"=w1211) -> ("error out"=w1213:errorcluster, "Port Out"=w1206:T5)  [unwired: 6 in]
              n552 = call "Check Idle.vi"("error in (no error)"=w1213, "Controller #"=w1209, "Port In"=w1206) -> ("error out (no error)"=w1212:errorcluster, "Port Out"=w1207:T6)  [unwired: 7 in]
            }
            frame True {
            }
          }
          n553 = property on="Graph" class="IntGraph (strict)"() -> ("XScale.Multiplier"=w1169:dbl)  [unwired: 2 in, 2 out]
          n554 = property on="Graph" class="IntGraph (strict)"() -> ("XScale.Offset"=w1170:dbl)  [unwired: 2 in, 2 out]
          n555 = property on="Graph" class="IntGraph (strict)"() -> ("YScale.Multiplier"=w1171:dbl)  [unwired: 2 in, 2 out]
          n556 = property on="Graph" class="IntGraph (strict)"() -> ("YScale.Offset"=w1172:dbl)  [unwired: 2 in, 2 out]
          n557 = Subtract(x=w1149, y=w1148) -> (x-y=w1147:u32)
          n558 = call "Max and Min Location.vi"("Array"=w1161, "x multiplier"=w1169, "x offset"=w1170, "y multiplier"=w1171, "y offset"=w1172) -> ("max value"=w1164:dbl, "Fast Axis Pos (Max)"=w1167:dbl, "Slow Axis Pos (Max)"=w1168:dbl, "min value"=w1166:dbl)  [unwired: 7 in]
          n559 = call "Time Left.vi"("Time Elapsed\nper slow"=w1147, "Current slow pos"=w1143, "Slow array size"=w1144) -> ("Estimated Time \nLeft"=w1145:dbl, "Percent Complete"=w1146:dbl)  [unwired: 7 in]
          n560 = flat-sequence {
            tunnel: w1155 -> [w1205]
            tunnel: w1156 -> [w1204]
            tunnel: w1157 -> [w1203]
            tunnel: w1160 -> [w1202]
            tunnel: w1154 -> [w1200]
            tunnel: [w1198] -> w1159
            frame #0 {
              n561 = call "Move rel mMc Edited.vi"("Controller #"=w1200, "rev dir?"=w1204, "Port In"=w1205, "error in (no error)"=w1202, "pos incr"=w1203) -> ("error out"=w1199:errorcluster, "Port Out"=w1201:T5)  [unwired: 5 in]
              n562 = call "Check Idle.vi"("error in (no error)"=w1199, "Controller #"=w1200, "Port In"=w1201) -> ("error out (no error)"=w1198:errorcluster)  [unwired: 7 in, 1 out]
            }
          }
          n563 = local write "Max Value"(w1164) -> ()
          n564 = local write "Fast Axis Pos\n(Max)"(w1167) -> ()
          n565 = local write "Slow Axis Pos\n(Max)"(w1168) -> ()
          n566 = local write "Estimated\nTime Left"(w1145) -> ()
          n567 = local write "Min Value"(w1166) -> ()
          n568 = local write "Percent Complete"(w1146) -> ()
        }
        n569 = call <vilib>:"DAQmx Clear Task.vi"("task in"=w1098) -> ()  [unwired: 14 in, 1 out]
      }
      frame "Angeled Scan" {
        n570 = Divide(x=w1313, y=w1311) -> (x/y=w1338:dbl)
        n571 = Divide(x=w1326, y=w1337) -> (x/y=w1339:dbl)
        n572 = Divide(x=w1326, y=2.0) -> (x/y=w1314:dbl)
        n573 = Divide(x=w1313, y=2.0) -> (x/y=w1322:dbl)
        n574 = Round Toward +Infinity(x=w1338) -> (ceil(x): smallest int >= x=w1310:dbl)
        n575 = Round Toward +Infinity(x=w1339) -> (ceil(x): smallest int >= x=w1303:dbl)
        n576 = call "Move rel mMc Edited.vi"("Controller #"=w1306, "rev dir?"=TRUE, "Port In"=w1312, "pos incr"=w1322) -> ("error out"=w1319:errorcluster, "Port Out"=w1320:T5)  [unwired: 6 in]
        n577 = call "Initialize DAQ Assistant.vi"("minimum value"=w1300, "maximum value"=w1301, "rate"=w1332, "number of samples"=w1329, "physical channels"=w1330) -> ("task out"=w1331:refnum<k21>)  [unwired: 5 in, 1 out]
        n578 = call "Move rel mMc Edited.vi"("Controller #"=w1309, "rev dir?"=TRUE, "Port In"=w1312, "pos incr"=w1314) -> ("error out"=w1324:errorcluster, "Port Out"=w1325:T5)  [unwired: 6 in]
        n579 = call "Check Idle (non scan).vi"("error in (no error)"=w1319, "Controller #"=w1306, "Port In"=w1320) -> ("Port Out"=w1317:T6)  [unwired: 7 in, 1 out]
        n580 = Increment(x=w1310) -> (x+1=w1335:dbl)
        n581 = Increment(x=w1303) -> (x+1=w1334:dbl)
        n582 = call "Check Idle (non scan).vi"("error in (no error)"=w1324, "Controller #"=w1309, "Port In"=w1325) -> ("Port Out"=w1316:T6)  [unwired: 7 in, 1 out]
        n583 = Initialize Array(-inf, w1335, w1334) -> (w1336:dbl[][])
        n584 = flat-sequence {
          tunnel: w1317 -> [w1342]
          tunnel: w1316 -> [_]
          tunnel: [w1342] -> w1315
          frame #0 {
          }
        }
        n585 = while {
          tunnel: w1306 -> [w1362]
          tunnel: w1309 -> [w1352]
          tunnel: w1315 -> [w1388]
          tunnel: w1337 -> [w1387]
          tunnel: w1326 -> [w1391]
          tunnel: w1311 -> [w1390]
          tunnel: w1313 -> [w1364]
          tunnel: w1312 -> [w1379]
          shift-right: [w1363] -> _
          shift-left: w1336 -> [w1383]
          tunnel: w1331 -> [w1377]
          tunnel: w1329 -> [w1376]
          tunnel: [w1365] -> w1302
          tunnel: w1309 -> [w1360]
          tunnel: w1308 -> [w1359]
          tunnel: w1307 -> [w1358]
          tunnel: w1306 -> [w1356]
          tunnel: w1305 -> [w1350]
          tunnel: w1304 -> [w1351]
          tunnel: w1303 -> [w1344]
          i -> [w1343]
          stop <- w1393 stop-if-true
          n586 = while {
            tunnel: w1362 -> [w1469]
            tunnel: w1388 -> [w1481]
            tunnel: w1390 -> [w1487]
            tunnel: w1364 -> [w1490]
            tunnel: [w1483] -> w1385
            tunnel: [w1489] -> w1389
            tunnel: w1343 -> [w1485]
            shift-right: [w1484] -> w1382
            shift-left: w1383 -> [w1486]
            tunnel: [w1482] -> w1361
            tunnel: [w1478] -> w1378
            tunnel: w1377 -> [w1477]
            tunnel: w1376 -> [w1476]
            tunnel: [w1476] -> w1375
            tunnel: w1360 -> [w1470]
            tunnel: w1359 -> [w1468]
            tunnel: w1358 -> [w1467]
            i -> [w1472]
            stop <- w1493 stop-if-true
            n587 = flat-sequence {
              tunnel: w1487 -> [w1520]
              tunnel: [w1519] -> w1488
              tunnel: w1480 -> [w1518]
              tunnel: [w1518] -> w1479
              frame #0 {
                n588 = local read "Abort Scan"() -> (w1522:bool)
                n589 = Select(t=0.0, s=w1522, f=w1520) -> (s? t:f=w1519:dbl)
              }
            }
            n590 = stacked-sequence {
              tunnel: w1488 -> [w1500 w1504 _]
              tunnel: w1469 -> [w1496 _ w1509]
              tunnel: w1481 -> [w1499 w1502 w1513]
              tunnel: w1479 -> [w1497 w1506 w1514]
              tunnel: [_ _ w1510] -> w1471
              tunnel: w1470 -> [_ w1503 w1508]
              tunnel: w1468 -> [w1494 _ _]
              tunnel: w1467 -> [_ w1501 _]
              frame #0 {
                n591 = Multiply(x=w1494, y=w1500) -> (x*y=w1495:dbl)
                n592 = call "Move rel mMc Edited.vi"("Controller #"=w1496, "rev dir?"=FALSE, "Port In"=w1499, "error in (no error)"=w1497, "pos incr"=w1495) -> ()  [unwired: 5 in, 2 out]
              }
              frame #1 {
                n593 = Multiply(x=w1501, y=w1504) -> (x*y=w1505:dbl)
                n594 = call "Move rel mMc Edited.vi"("Controller #"=w1503, "rev dir?"=FALSE, "Port In"=w1502, "error in (no error)"=w1506, "pos incr"=w1505) -> ()  [unwired: 5 in, 2 out]
              }
              frame #2 {
                n595 = call "Check Idle.vi"("error in (no error)"=w1514, "Controller #"=w1509, "Port In"=w1513) -> ("error out (no error)"=w1511:errorcluster, "Port Out"=w1512:T6)  [unwired: 7 in]
                n596 = call "Check Idle.vi"("error in (no error)"=w1511, "Controller #"=w1508, "Port In"=w1512) -> ("error out (no error)"=w1510:errorcluster)  [unwired: 7 in, 1 out]
              }
            }
            n597 = flat-sequence {
              tunnel: w1486 -> [w1537]
              tunnel: w1485 -> [w1535]
              tunnel: w1472 -> [w1536]
              tunnel: [w1533] -> w1484
              tunnel: [w1530] -> w1480
              tunnel: [w1532] -> w1478
              tunnel: w1477 -> [w1531]
              tunnel: w1476 -> [w1529]
              frame #0 {
                n598 = call "Measure and Update Array.vi"("Array In"=w1537, "number of samples per channel"=w1529, "task/channels in"=w1531, "Row"=w1536, "Column"=w1535, "Invert?"=FALSE) -> ("Array Out"=w1533:dbl[][], "task out"=w1532:refnum<k21>, "Measurement"=w1528:dbl, "error out"=w1530:errorcluster)  [unwired: 6 in]
                n599 = local write "Measured"(w1528) -> ()
                n600 = local write "Graph"(w1533) -> ()
              }
            }
            n601 = Increment(x=w1472) -> (x+1=w1492:i32)
            n602 = Tick Count (ms)() -> (millisecond timer value=w1475:u32)
            n603 = Multiply(x=w1487, y=w1492) -> (x*y=w1489:dbl)
            n604 = flat-sequence {
              tunnel: w1475 -> [w1517]
              tunnel: w1474 -> [w1516]
              tunnel: [w1515] -> w1473
              frame #0 {
                n605 = Subtract(x=w1516, y=w1517) -> (x-y=w1515:u32)
              }
            }
            n606 = Greater Or Equal?(x=w1489, y=w1490) -> (x >= y?=w1491:bool)
            n607 = flat-sequence {
              tunnel: [w1527] -> w1493
              tunnel: w1491 -> [w1526]
              tunnel: w1471 -> [w1525]
              tunnel: [w1525] -> w1483
              tunnel: [w1523] -> w1474
              frame #0 {
                n608 = local read "Abort Scan"() -> (w1524:bool)
                n609 = Tick Count (ms)() -> (millisecond timer value=w1523:u32)
                n610 = Or(x=w1526, y=w1524) -> (x .or. y?=w1527:bool)
              }
            }
            n611 = Increment(x=w1472) -> (x+1=w1482:i32)
            n612 = local write "Time per Pixel"(w1473) -> ()
          }
          n613 = Multiply(x=w1387, y=w1343) -> (x*y=w1392:dbl)
          n614 = Greater Or Equal?(x=w1392, y=w1391) -> (x >= y?=w1380:bool)
          n615 = Tick Count (ms)() -> (millisecond timer value=w1348:u32)
          n616 = flat-sequence {
            tunnel: w1389 -> [w1450]
            tunnel: [w1449] -> w1353
            frame #0 {
              n617 = local read "Abort Scan"() -> (w1452:bool)
              n618 = Select(t=0.0, s=w1452, f=w1450) -> (s? t:f=w1449:dbl)
            }
          }
          n619 = flat-sequence {
            tunnel: w1385 -> [w1456]
            tunnel: [w1455] -> w1354
            tunnel: w1382 -> [w1462]
            tunnel: w1343 -> [w1460]
            tunnel: w1361 -> [w1461]
            tunnel: [w1458] -> w1363
            tunnel: w1378 -> [w1457]
            tunnel: [w1454] -> w1365
            tunnel: w1375 -> [w1453]
            frame #0 {
              n620 = call "Measure and Update Array.vi"("Array In"=w1462, "number of samples per channel"=w1453, "task/channels in"=w1457, "Row"=w1461, "Column"=w1460, "error in"=w1456, "Invert?"=FALSE) -> ("Array Out"=w1458:dbl[][], "task out"=w1454:refnum<k21>, "error out"=w1455:errorcluster)  [unwired: 5 in, 1 out]
              n621 = local write "Graph"(w1458) -> ()
            }
          }
          n622 = flat-sequence {
            tunnel: w1387 -> [w1446]
            tunnel: [w1445] -> w1384
            tunnel: w1386 -> [w1444]
            tunnel: [w1444] -> w1381
            frame #0 {
              n623 = local read "Back scan delay"() -> (w1443:u32)
              n624 = local read "Abort Scan"() -> (w1448:bool)
              n625 = Select(t=0.0, s=w1448, f=w1446) -> (s? t:f=w1445:dbl)
              n626 = Wait (ms)(milliseconds to wait=w1443) -> ()  [unwired: 1 out]
            }
          }
          n627 = stacked-sequence {
            tunnel: w1354 -> [w1400 w1407 w1411]
            tunnel: w1353 -> [w1396 w1404 _]
            tunnel: [_ _ w1408] -> w1386
            tunnel: w1379 -> [w1399 w1406 w1414]
            tunnel: [_ _ w1412] -> w1367
            tunnel: w1362 -> [w1398 _ w1410]
            tunnel: TRUE ("rev dir?") -> [w1397 w1405 _]
            tunnel: w1352 -> [_ w1402 w1409]
            tunnel: w1351 -> [_ w1401 _]
            tunnel: w1350 -> [w1394 _ _]
            frame #0 {
              n628 = Multiply(x=w1396, y=w1394) -> (x*y=w1395:dbl)
              n629 = call "Move rel mMc Edited.vi"("Controller #"=w1398, "rev dir?"=w1397, "Port In"=w1399, "error in (no error)"=w1400, "pos incr"=w1395) -> ()  [unwired: 5 in, 2 out]
            }
            frame #1 {
              n630 = Multiply(x=w1404, y=w1401) -> (x*y=w1403:dbl)
              n631 = call "Move rel mMc Edited.vi"("Controller #"=w1402, "rev dir?"=w1405, "Port In"=w1406, "error in (no error)"=w1407, "pos incr"=w1403) -> ()  [unwired: 5 in, 2 out]
            }
            frame #2 {
              n632 = call "Check Idle.vi"("error in (no error)"=w1411, "Controller #"=w1410, "Port In"=w1414) -> ("Port Out"=w1413:T6)  [unwired: 7 in, 1 out]
              n633 = call "Check Idle.vi"("Controller #"=w1409, "Port In"=w1413) -> ("error out (no error)"=w1408:errorcluster, "Port Out"=w1412:T6)  [unwired: 8 in]
            }
          }
          n634 = flat-sequence {
            tunnel: [w1466] -> w1393
            tunnel: w1380 -> [w1465]
            tunnel: w1357 -> [_]
            tunnel: [w1463] -> w1349
            frame #0 {
              n635 = local read "Abort Scan"() -> (w1464:bool)
              n636 = Tick Count (ms)() -> (millisecond timer value=w1463:u32)
              n637 = Or(x=w1465, y=w1464) -> (x .or. y?=w1466:bool)
            }
          }
          n638 = property on="Graph" class="IntGraph (strict)"() -> ("XScale.Multiplier"=w1371:dbl)  [unwired: 2 in, 2 out]
          n639 = property on="Graph" class="IntGraph (strict)"() -> ("XScale.Offset"=w1372:dbl)  [unwired: 2 in, 2 out]
          n640 = property on="Graph" class="IntGraph (strict)"() -> ("YScale.Multiplier"=w1373:dbl)  [unwired: 2 in, 2 out]
          n641 = property on="Graph" class="IntGraph (strict)"() -> ("YScale.Offset"=w1374:dbl)  [unwired: 2 in, 2 out]
          n642 = case shown="False" w1380 {
            tunnel: [w1422 w1442] -> w1357
            tunnel: w1384 -> [w1421 _]
            tunnel: w1381 -> [w1420 w1442]
            tunnel: w1352 -> [w1419 _]
            tunnel: w1367 -> [w1418 _]
            tunnel: w1356 -> [w1417 _]
            tunnel: w1351 -> [w1416 _]
            tunnel: w1350 -> [w1415 _]
            frame False {
              n643 = stacked-sequence {
                tunnel: [_ _ w1439] -> w1422
                tunnel: w1421 -> [w1428 w1430 _]
                tunnel: w1420 -> [w1427 w1434 w1441]
                tunnel: w1419 -> [w1426 _ w1436]
                tunnel: w1418 -> [w1425 w1433 w1438]
                tunnel: w1417 -> [_ w1432 w1435]
                tunnel: w1416 -> [w1423 _ _]
                tunnel: w1415 -> [_ w1429 _]
                frame #0 {
                  n644 = Multiply(x=w1428, y=w1423) -> (x*y=w1424:dbl)
                  n645 = call "Move rel mMc Edited.vi"("Controller #"=w1426, "Port In"=w1425, "error in (no error)"=w1427, "pos incr"=w1424) -> ()  [unwired: 6 in, 2 out]
                }
                frame #1 {
                  n646 = Multiply(x=w1430, y=w1429) -> (x*y=w1431:dbl)
                  n647 = call "Move rel mMc Edited.vi"("Controller #"=w1432, "Port In"=w1433, "error in (no error)"=w1434, "pos incr"=w1431) -> ()  [unwired: 6 in, 2 out]
                }
                frame #2 {
                  n648 = call "Check Idle.vi"("error in (no error)"=w1441, "Controller #"=w1436, "Port In"=w1438) -> ("error out (no error)"=w1440:errorcluster, "Port Out"=w1437:T6)  [unwired: 7 in]
                  n649 = call "Check Idle.vi"("error in (no error)"=w1440, "Controller #"=w1435, "Port In"=w1437) -> ("error out (no error)"=w1439:errorcluster)  [unwired: 7 in, 1 out]
                }
              }
            }
            frame True {
            }
          }
          n650 = Subtract(x=w1349, y=w1348) -> (x-y=w1347:u32)
          n651 = call "Max and Min Location.vi"("Array"=w1363, "x multiplier"=w1371, "x offset"=w1372, "y multiplier"=w1373, "y offset"=w1374) -> ("max value"=w1366:dbl, "Fast Axis Pos (Max)"=w1369:dbl, "Slow Axis Pos (Max)"=w1370:dbl, "min value"=w1368:dbl)  [unwired: 7 in]
          n652 = call "Time Left.vi"("Time Elapsed\nper slow"=w1347, "Current slow pos"=w1343, "Slow array size"=w1344) -> ("Estimated Time \nLeft"=w1345:dbl, "Percent Complete"=w1346:dbl)  [unwired: 7 in]
          n653 = local write "Max Value"(w1366) -> ()
          n654 = local write "Slow Axis Pos\n(Max)"(w1370) -> ()
          n655 = local write "Fast Axis Pos\n(Max)"(w1369) -> ()
          n656 = local write "Estimated\nTime Left"(w1345) -> ()
          n657 = local write "Min Value"(w1368) -> ()
          n658 = local write "Percent Complete"(w1346) -> ()
        }
        n659 = call <vilib>:"DAQmx Clear Task.vi"("task in"=w1302) -> ()  [unwired: 14 in, 1 out]
      }
      frame "Angeled Line Scan" {
        n660 = flat-sequence {
          tunnel: w1565 -> [w1613]
          tunnel: w1565 -> [w1618]
          tunnel: w1565 -> [w1617]
          tunnel: w1559 -> [w1616]
          tunnel: w1544 -> [w1615]
          tunnel: w1558 -> [w1614]
          tunnel: "X" -> [w1610]
          tunnel: "Y" -> [w1611]
          tunnel: "Z" -> [w1612]
          tunnel: [w1613] -> w1555
          tunnel: [w1612] -> w1553
          tunnel: [w1611] -> w1552
          tunnel: [w1610] -> w1551
          tunnel: w1540 -> [w1609]
          tunnel: w1550 -> [w1606]
          tunnel: w1549 -> [w1605]
          tunnel: w1555 -> [w1619]
          tunnel: w1553 -> [w1622]
          tunnel: w1552 -> [w1621]
          tunnel: w1551 -> [w1620]
          frame #0 {
            n661 = Not(x=w1609) -> (.not. x?=w1608:bool)
            n662 = call "Move rel mMc Edited.vi"("Controller #"=w1610, "rev dir?"=w1608, "Port In"=w1617, "pos incr"=w1616) -> ()  [unwired: 6 in, 2 out]
            n663 = Not(x=w1606) -> (.not. x?=w1607:bool)
            n664 = call "Move rel mMc Edited.vi"("Controller #"=w1611, "rev dir?"=w1607, "Port In"=w1618, "pos incr"=w1615) -> ()  [unwired: 6 in, 2 out]
            n665 = Not(x=w1605) -> (.not. x?=w1604:bool)
            n666 = call "Move rel mMc Edited.vi"("Controller #"=w1612, "rev dir?"=w1604, "Port In"=w1613, "pos incr"=w1614) -> ()  [unwired: 6 in, 2 out]
          }
          frame #1 {
            n667 = call "Check Idle.vi"("Controller #"=w1620, "Port In"=w1619) -> ()  [unwired: 8 in, 2 out]
            n668 = call "Check Idle.vi"("Controller #"=w1621, "Port In"=w1619) -> ()  [unwired: 8 in, 2 out]
            n669 = call "Check Idle.vi"("Controller #"=w1622, "Port In"=w1619) -> ()  [unwired: 8 in, 2 out]
          }
        }
        n670 = call "Initialize DAQ Assistant.vi"("minimum value"=w1538, "maximum value"=w1539, "rate"=w1589, "number of samples"=w1568, "physical channels"=w1590) -> ("task out"=w1588:refnum<k21>)  [unwired: 5 in, 1 out]
        n671 = Divide(x="phi", y=180.0) -> (x/y=w1598:dbl)
        n672 = Divide(x="theta", y=180.0) -> (x/y=w1603:dbl)
        n673 = Multiply(x=w1598, y=3.141592653589793) -> (x*y=w1594:dbl)
        n674 = Multiply(x=w1603, y=3.141592653589793) -> (x*y=w1599:dbl)
        n675 = Divide(x="rho Step Size (microns)", y=1000.0 ("x")) -> (x/y=w1570:dbl)
        n676 = Sine & Cosine(0:w1594) -> (1:w1585:dbl, 2:w1587:dbl)
        n677 = Sine & Cosine(0:w1599) -> (1:w1586:dbl, 2:w1548:dbl)
        n678 = Multiply(x=w1586, y=w1585) -> (x*y=w1547:dbl)
        n679 = Multiply(x=w1586, y=w1587) -> (x*y=w1546:dbl)
        n680 = Multiply(x=w1546, y=w1570) -> (x*y=w1583:dbl)
        n681 = Multiply(x=w1547, y=w1570) -> (x*y=w1579:dbl)
        n682 = Multiply(x=w1548, y=w1570) -> (x*y=w1580:dbl)
        n683 = property on="Waveform Graph" class="WFGraph (strict)"("XScale.Multiplier"=w1570) -> ()  [unwired: 2 in, 2 out]
        n684 = Divide(x="rho Length (microns)", y=1000.0) -> (x/y=w1564:dbl)
        n685 = Greater Than 0?(x=w1583) -> (x > 0?=w1584:bool)
        n686 = Greater Than 0?(x=w1579) -> (x > 0?=w1581:bool)
        n687 = Greater Than 0?(x=w1580) -> (x > 0?=w1582:bool)
        n688 = Absolute Value(x=w1548) -> (abs(x)=w1541:dbl)
        n689 = Absolute Value(x=w1546) -> (abs(x)=w1542:dbl)
        n690 = Absolute Value(x=w1547) -> (abs(x)=w1543:dbl)
        n691 = Divide(x=w1564, y=w1570) -> (x/y=w1574:dbl)
        n692 = Absolute Value(x=w1580) -> (abs(x)=w1561:dbl)
        n693 = case shown="False" w1584 {
          tunnel: [TRUE FALSE] -> w1540
          frame False {
          }
          frame True {
          }
        }
        n694 = case shown="False" w1581 {
          tunnel: [TRUE FALSE] -> w1550
          frame False {
          }
          frame True {
          }
        }
        n695 = case shown="False" w1582 {
          tunnel: [TRUE FALSE] -> w1549
          frame False {
          }
          frame True {
          }
        }
        n696 = Absolute Value(x=w1583) -> (abs(x)=w1545:dbl)
        n697 = Absolute Value(x=w1579) -> (abs(x)=w1560:dbl)
        n698 = Round Toward +Infinity(x=w1574) -> (ceil(x): smallest int >= x=w1573:dbl)
        n699 = Increment(x=w1573) -> (x+1=w1572:dbl)
        n700 = Divide(x=w1564, y=2.0) -> (x/y=w1562:dbl)
        n701 = Multiply(x=w1562, y=w1542) -> (x*y=w1559:dbl)
        n702 = Multiply(x=w1562, y=w1543) -> (x*y=w1544:dbl)
        n703 = Initialize Array(-inf, w1572) -> (w1571:dbl[])
        n704 = Multiply(x=w1562, y=w1541) -> (x*y=w1558:dbl)
        n705 = while {
          tunnel: "X" -> [w1650]
          tunnel: "Y" -> [w1649]
          tunnel: "Z" -> [w1648]
          tunnel: w1565 -> [w1641]
          tunnel: [w1641] -> w1593
          tunnel: w1588 -> [w1644]
          tunnel: w1568 -> [w1643]
          tunnel: w1545 -> [w1642]
          tunnel: w1540 -> [w1640]
          tunnel: w1560 -> [w1639]
          tunnel: w1561 -> [w1638]
          tunnel: w1550 -> [w1637]
          tunnel: w1549 -> [w1636]
          tunnel: w1570 -> [w1635]
          tunnel: w1564 -> [w1632]
          shift-right: [w1627] -> _
          shift-left: w1571 -> [w1625]
          tunnel: [w1626] -> w1567
          i -> [w1634]
          stop <- w1630 stop-if-true
          n706 = call "Move rel mMc Edited.vi"("Controller #"=w1650, "rev dir?"=w1640, "Port In"=w1641, "pos incr"=w1642) -> ("error out"=w1651:errorcluster)  [unwired: 6 in, 1 out]
          n707 = call "Move rel mMc Edited.vi"("Controller #"=w1649, "rev dir?"=w1637, "Port In"=w1641, "pos incr"=w1639) -> ("error out"=w1652:errorcluster)  [unwired: 6 in, 1 out]
          n708 = call "Move rel mMc Edited.vi"("Controller #"=w1648, "rev dir?"=w1636, "Port In"=w1641, "pos incr"=w1638) -> ("error out"=w1653:errorcluster)  [unwired: 6 in, 1 out]
          n709 = flat-sequence {
            tunnel: w1653 -> [_]
            tunnel: w1652 -> [_]
            tunnel: w1651 -> [_]
            tunnel: w1650 -> [w1672]
            tunnel: w1649 -> [w1671]
            tunnel: w1648 -> [w1670]
            tunnel: [w1669] -> w1647
            tunnel: [w1668] -> w1646
            tunnel: [w1667] -> w1645
            tunnel: w1641 -> [w1666]
            frame #0 {
              n710 = call "Check Idle.vi"("Controller #"=w1671, "Port In"=w1666) -> ("error out (no error)"=w1668:errorcluster)  [unwired: 8 in, 1 out]
              n711 = call "Check Idle.vi"("Controller #"=w1670, "Port In"=w1666) -> ("error out (no error)"=w1669:errorcluster)  [unwired: 8 in, 1 out]
              n712 = call "Check Idle.vi"("Controller #"=w1672, "Port In"=w1666) -> ("error out (no error)"=w1667:errorcluster)  [unwired: 8 in, 1 out]
            }
          }
          n713 = Increment(x=w1634) -> (x+1=w1628:i32)
          n714 = Multiply(x=w1635, y=w1628) -> (x*y=w1633:dbl)
          n715 = Greater?(x=w1633, y=w1632) -> (0:w1631:bool)
          n716 = flat-sequence {
            tunnel: w1647 -> [_]
            tunnel: w1646 -> [_]
            tunnel: w1645 -> [w1664]
            tunnel: w1644 -> [w1662]
            tunnel: w1643 -> [w1661]
            tunnel: [w1665] -> w1629
            tunnel: w1628 -> [w1663]
            tunnel: [w1660] -> w1627
            tunnel: [w1658] -> w1626
            tunnel: w1625 -> [w1657]
            frame #0 {
              n717 = call "Measure Line Scan.vi"("number of samples per channel"=w1661, "error in"=w1664, "Iterator"=w1663, "task/channels in"=w1662, "Array in"=w1657) -> ("error out"=w1665:errorcluster, "mean"=→"Current Volts":dbl, "task out"=w1658:refnum<k21>, "Array out"=w1660:dbl[])  [unwired: 3 in]
              "Waveform Graph" <- w1660
            }
          }
          n718 = flat-sequence {
            tunnel: w1631 -> [w1656]
            tunnel: [w1655] -> w1630
            tunnel: w1629 -> [_]
            frame #0 {
              n719 = local read "Abort Scan"() -> (w1654:bool)
              n720 = Or(x=w1654, y=w1656) -> (x .or. y?=w1655:bool)
            }
          }
        }
        n721 = flat-sequence {
          tunnel: w1567 -> [w1623]
          tunnel: ["Move to Origin (ALS)" ("Scan Type")] -> w1566
          frame #0 {
            n722 = call <vilib>:"DAQmx Clear Task.vi"("task in"=w1623) -> ()  [unwired: 14 in, 1 out]
          }
        }
      }
      frame "Move to Origin" {
        w1687 = "3" ("Controller #")
        w1688 = "2" ("Controller #")
        w1689 = "1" ("Controller #")
        n723 = local read "Scan Origin"() -> (w1696:T1)
        n724 = Unbundle By Name(w1696) -> ("Cnt pos 1"=w1692:dbl, "Cnt pos 2"=w1691:dbl, "Cnt pos 3"=w1690:dbl)
        n725 = call "Move abs mMc.vi"("target pos in"=w1692, "Port"=w1686, "Controller #"=w1689) -> ("error out"=w1695:errorcluster)  [unwired: 6 in]
        n726 = call "Move abs mMc.vi"("target pos in"=w1691, "Port"=w1686, "Controller #"=w1688) -> ("error out"=w1694:errorcluster)  [unwired: 6 in]
        n727 = call "Move abs mMc.vi"("target pos in"=w1690, "Port"=w1686, "Controller #"=w1687) -> ("error out"=w1693:errorcluster)  [unwired: 6 in]
        n728 = call "Check Idle (non scan).vi"("error in (no error)"=w1695, "Controller #"=w1689, "Port In"=w1686) -> ("Port Out"=w1682:T6)  [unwired: 7 in, 1 out]
        n729 = call "Check Idle (non scan).vi"("error in (no error)"=w1694, "Controller #"=w1688, "Port In"=w1686) -> ("Port Out"=w1681:T6)  [unwired: 7 in, 1 out]
        n730 = call "Check Idle (non scan).vi"("error in (no error)"=w1693, "Controller #"=w1687, "Port In"=w1686) -> ("Port Out"=w1680:T6)  [unwired: 7 in, 1 out]
        n731 = flat-sequence {
          tunnel: w1682 -> [w1697]
          tunnel: w1681 -> [_]
          tunnel: w1680 -> [_]
          tunnel: [w1697] -> w1679
          frame #0 {
          }
        }
      }
      frame "Move to Origin (ALS)" {
        w1707 = "3" ("Controller #")
        w1708 = "2" ("Controller #")
        w1709 = "1" ("Controller #")
        n732 = local read "Scan Origin (ALS)"() -> (w1698:T1)
        n733 = Unbundle By Name(w1698) -> ("Cnt pos 1"=w1712:dbl, "Cnt pos 2"=w1711:dbl, "Cnt pos 3"=w1710:dbl)
        n734 = call "Move abs mMc.vi"("target pos in"=w1712, "Port"=w1706, "Controller #"=w1709) -> ("error out"=w1715:errorcluster)  [unwired: 6 in]
        n735 = call "Move abs mMc.vi"("target pos in"=w1711, "Port"=w1706, "Controller #"=w1708) -> ("error out"=w1714:errorcluster)  [unwired: 6 in]
        n736 = call "Move abs mMc.vi"("target pos in"=w1710, "Port"=w1706, "Controller #"=w1707) -> ("error out"=w1713:errorcluster)  [unwired: 6 in]
        n737 = call "Check Idle (non scan).vi"("error in (no error)"=w1715, "Controller #"=w1709, "Port In"=w1706) -> ("Port Out"=w1702:T6)  [unwired: 7 in, 1 out]
        n738 = call "Check Idle (non scan).vi"("error in (no error)"=w1714, "Controller #"=w1708, "Port In"=w1706) -> ("Port Out"=w1701:T6)  [unwired: 7 in, 1 out]
        n739 = call "Check Idle (non scan).vi"("error in (no error)"=w1713, "Controller #"=w1707, "Port In"=w1706) -> ("Port Out"=w1700:T6)  [unwired: 7 in, 1 out]
        n740 = flat-sequence {
          tunnel: w1702 -> [w1716]
          tunnel: w1701 -> [_]
          tunnel: w1700 -> [_]
          tunnel: [w1716] -> w1699
          frame #0 {
          }
        }
      }
      frame "Move to Cursor 1" {
        n741 = property on="Graph" class="IntGraph (strict)"("Active Cursor"=u32 0) -> (error out=w1719:errorcluster)  [unwired: 2 in, 1 out]
        n742 = property on="Graph" class="IntGraph (strict)"(error in=w1719) -> ("Cursor.Cursor Position"=w1718:T7)  [unwired: 1 in, 2 out]
        n743 = Unbundle By Name(w1718) -> ("Cursor X"=w1730:dbl, "Cursor Y"=w1729:dbl)
        n744 = call "Move abs mMc.vi"("target pos in"=w1730, "Port"=w1728, "Controller #"=w1727) -> ("error out"=w1725:errorcluster)  [unwired: 6 in]
        n745 = call "Check Idle (non scan).vi"("error in (no error)"=w1725, "Controller #"=w1727, "Port In"=w1728) -> ("Port Out"=w1722:T6)  [unwired: 7 in, 1 out]
        n746 = call "Move abs mMc.vi"("target pos in"=w1729, "Port"=w1728, "error in (no error)"=w1725, "Controller #"=w1726) -> ("error out"=w1724:errorcluster)  [unwired: 5 in]
        n747 = call "Check Idle (non scan).vi"("error in (no error)"=w1724, "Controller #"=w1726, "Port In"=w1728) -> ("Port Out"=w1721:T6)  [unwired: 7 in, 1 out]
        n748 = flat-sequence {
          tunnel: w1722 -> [_]
          tunnel: w1721 -> [w1733]
          tunnel: [w1733] -> w1720
          frame #0 {
          }
        }
      }
      frame "Move to Cursor 2" {
        n749 = property on="Graph" class="IntGraph (strict)"("Active Cursor"=u32 1) -> (error out=w1736:errorcluster)  [unwired: 2 in, 1 out]
        n750 = property on="Graph" class="IntGraph (strict)"(error in=w1736) -> ("Cursor.Cursor Position"=w1735:T7)  [unwired: 1 in, 2 out]
        n751 = Unbundle By Name(w1735) -> ("Cursor X"=w1747:dbl, "Cursor Y"=w1746:dbl)
        n752 = call "Move abs mMc.vi"("target pos in"=w1747, "Port"=w1745, "Controller #"=w1744) -> ("error out"=w1742:errorcluster)  [unwired: 6 in]
        n753 = call "Check Idle (non scan).vi"("error in (no error)"=w1742, "Controller #"=w1744, "Port In"=w1745) -> ("Port Out"=w1738:T6)  [unwired: 7 in, 1 out]
        n754 = call "Move abs mMc.vi"("target pos in"=w1746, "Port"=w1745, "error in (no error)"=w1742, "Controller #"=w1743) -> ("error out"=w1741:errorcluster)  [unwired: 5 in]
        n755 = call "Check Idle (non scan).vi"("error in (no error)"=w1741, "Controller #"=w1743, "Port In"=w1745) -> ("Port Out"=w1739:T6)  [unwired: 7 in, 1 out]
        n756 = flat-sequence {
          tunnel: w1739 -> [w1750]
          tunnel: [w1750] -> w1737
          tunnel: w1738 -> [_]
          frame #0 {
          }
        }
      }
      frame "Move to rho" {
        # "z"
        # "y"
        # "x"
        n757 = property on="Waveform Graph" class="WFGraph (strict)"() -> ("Cursor.Cursor X"=w1764:dbl)  [unwired: 2 in, 2 out]
        n758 = local read "phi"() -> (w1785:dbl)
        n759 = local read "theta"() -> (w1786:dbl)
        n760 = Divide(x=w1785, y=180.0) -> (x/y=w1793:dbl)
        n761 = local read "rho Length (microns)"() -> (w1768:dbl)
        n762 = Divide(x=w1786, y=180.0) -> (x/y=w1797:dbl)
        n763 = Multiply(x=w1793, y=3.141592653589793) -> (x*y=w1790:dbl)
        n764 = Multiply(x=w1797, y=3.141592653589793) -> (x*y=w1794:dbl)
        n765 = Sine & Cosine(0:w1790) -> (1:w1787:dbl, 2:w1789:dbl)
        n766 = Sine & Cosine(0:w1794) -> (1:w1788:dbl, 2:w1761:dbl)
        n767 = Multiply(x=w1788, y=w1787) -> (x*y=w1762:dbl)
        n768 = Multiply(x=w1788, y=w1789) -> (x*y=w1763:dbl)
        n769 = Divide(x=w1768, y=1000.0) -> (x/y=w1766:dbl)
        n770 = Multiply(x=w1762, y=w1764) -> (x*y=w1756:dbl)
        n771 = Multiply(x=w1761, y=w1764) -> (x*y=w1753:dbl)
        n772 = Multiply(x=w1763, y=w1764) -> (x*y=w1758:dbl)
        n773 = Divide(x=w1766, y=2.0) -> (x/y=w1760:dbl)
        n774 = Multiply(x=w1763, y=w1760) -> (x*y=w1759:dbl)
        n775 = Multiply(x=w1762, y=w1760) -> (x*y=w1755:dbl)
        n776 = Multiply(x=w1761, y=w1760) -> (x*y=w1751:dbl)
        n777 = Subtract(x=w1758, y=w1759) -> (x-y=w1757:dbl)
        n778 = Subtract(x=w1756, y=w1755) -> (x-y=w1754:dbl)
        n779 = local read "X"() -> (w1771:string)
        n780 = local read "Y"() -> (w1770:string)
        n781 = local read "Z"() -> (w1769:string)
        n782 = Subtract(x=w1753, y=w1751) -> (x-y=w1752:dbl)
        n783 = case shown="\"1\", Default" w1771 {
          tunnel: [w1820 w1822 w1824] -> w1781
          frame "1", Default {
            n784 = local read "Scan Origin (ALS)"() -> (w1819:T1)
            n785 = Unbundle By Name(w1819) -> ("Cnt pos 1"=w1820:dbl)  [unwired: 2 out]
          }
          frame "2" {
            n786 = local read "Scan Origin (ALS)"() -> (w1821:T1)
            n787 = Unbundle By Name(w1821) -> ("Cnt pos 2"=w1822:dbl)  [unwired: 2 out]
          }
          frame "3" {
            n788 = local read "Scan Origin (ALS)"() -> (w1823:T1)
            n789 = Unbundle By Name(w1823) -> ("Cnt pos 3"=w1824:dbl)  [unwired: 2 out]
          }
        }
        n790 = case shown="\"2\", Default" w1770 {
          tunnel: [w1814 w1816 w1818] -> w1780
          frame "1" {
            n791 = local read "Scan Origin (ALS)"() -> (w1813:T1)
            n792 = Unbundle By Name(w1813) -> ("Cnt pos 1"=w1814:dbl)  [unwired: 2 out]
          }
          frame "2", Default {
            n793 = local read "Scan Origin (ALS)"() -> (w1815:T1)
            n794 = Unbundle By Name(w1815) -> ("Cnt pos 2"=w1816:dbl)  [unwired: 2 out]
          }
          frame "3" {
            n795 = local read "Scan Origin (ALS)"() -> (w1817:T1)
            n796 = Unbundle By Name(w1817) -> ("Cnt pos 3"=w1818:dbl)  [unwired: 2 out]
          }
        }
        n797 = case shown="\"3\", Default" w1769 {
          tunnel: [w1808 w1810 w1812] -> w1779
          frame "1" {
            n798 = local read "Scan Origin (ALS)"() -> (w1807:T1)
            n799 = Unbundle By Name(w1807) -> ("Cnt pos 1"=w1808:dbl)  [unwired: 2 out]
          }
          frame "2" {
            n800 = local read "Scan Origin (ALS)"() -> (w1809:T1)
            n801 = Unbundle By Name(w1809) -> ("Cnt pos 2"=w1810:dbl)  [unwired: 2 out]
          }
          frame "3", Default {
            n802 = local read "Scan Origin (ALS)"() -> (w1811:T1)
            n803 = Unbundle By Name(w1811) -> ("Cnt pos 3"=w1812:dbl)  [unwired: 2 out]
          }
        }
        n804 = Add(x=w1780, y=w1754) -> (x+y=w1777:dbl)
        n805 = Add(x=w1781, y=w1757) -> (x+y=w1778:dbl)
        n806 = Add(x=w1779, y=w1752) -> (x+y=w1776:dbl)
        n807 = call "Move abs mMc.vi"("target pos in"=w1778, "Port"=w1775, "Controller #"=w1771) -> ("error out"=w1772:errorcluster)  [unwired: 6 in]
        n808 = call "Move abs mMc.vi"("target pos in"=w1777, "Port"=w1775, "Controller #"=w1770) -> ("error out"=w1773:errorcluster)  [unwired: 6 in]
        n809 = call "Move abs mMc.vi"("target pos in"=w1776, "Port"=w1775, "Controller #"=w1769) -> ("error out"=w1774:errorcluster)  [unwired: 6 in]
        n810 = flat-sequence {
          tunnel: w1775 -> [w1806]
          tunnel: w1775 -> [w1805]
          tunnel: w1775 -> [w1804]
          tunnel: w1774 -> [w1803]
          tunnel: w1773 -> [w1802]
          tunnel: w1772 -> [w1801]
          tunnel: w1771 -> [w1800]
          tunnel: w1770 -> [w1799]
          tunnel: w1769 -> [w1798]
          frame #0 {
            n811 = call "Check Idle (non scan).vi"("error in (no error)"=w1803, "Controller #"=w1798, "Port In"=w1804) -> ()  [unwired: 7 in, 2 out]
            n812 = call "Check Idle (non scan).vi"("error in (no error)"=w1802, "Controller #"=w1799, "Port In"=w1805) -> ()  [unwired: 7 in, 2 out]
            n813 = call "Check Idle (non scan).vi"("error in (no error)"=w1801, "Controller #"=w1800, "Port In"=w1806) -> ()  [unwired: 7 in, 2 out]
          }
        }
      }
      frame "Move to Max Value Position" {
        n814 = local read "Fast Axis Pos\n(Max)"() -> (w1836:dbl)
        n815 = call "Move abs mMc.vi"("target pos in"=w1836, "Port"=w1834, "Controller #"=w1833) -> ("error out"=w1831:errorcluster)  [unwired: 6 in]
        n816 = call "Check Idle (non scan).vi"("error in (no error)"=w1831, "Controller #"=w1833, "Port In"=w1834) -> ("Port Out"=w1829:T6)  [unwired: 7 in, 1 out]
        n817 = local read "Slow Axis Pos\n(Max)"() -> (w1835:dbl)
        n818 = call "Move abs mMc.vi"("target pos in"=w1835, "Port"=w1834, "Controller #"=w1832) -> ("error out"=w1830:errorcluster)  [unwired: 6 in]
        n819 = call "Check Idle (non scan).vi"("error in (no error)"=w1830, "Controller #"=w1832, "Port In"=w1834) -> ("Port Out"=w1828:T6)  [unwired: 7 in, 1 out]
        n820 = flat-sequence {
          tunnel: w1829 -> [w1838]
          tunnel: w1828 -> [_]
          tunnel: [w1838] -> w1827
          frame #0 {
          }
        }
      }
      frame "Export Data" {
        n821 = invoke on="Graph" class="IntGraph (strict)" method="Export Data to Excel"() -> ()  [unwired: 3 in, 3 out]
      }
      frame "Save Image" {
        n822 = local read "Save Intensity Graph"() -> (w1843:bool)
        n823 = case shown="False" w1843 {
          frame False {
            n824 = property on="Waveform Graph" class="WFGraph (strict)"() -> ("CrsrList"=w1852:T8)  [unwired: 2 in, 2 out]
            n825 = Array Size(array=w1852) -> (size(s)=w1859:i32)
            n826 = for {
              N: w1859 -> [_]
              tunnel: [w1864] -> w1853
              i -> [w1865]
              n827 = property on="Waveform Graph" class="WFGraph (strict)"("Active Cursor"=w1865) -> (error out=w1866:errorcluster)  [unwired: 2 in, 1 out]
              n828 = property on="Waveform Graph" class="WFGraph (strict)"(error in=w1866, "Cursor.Visible"=FALSE) -> (error out=w1864:errorcluster)  [unwired: 1 in, 1 out]
            }
            n829 = property on="Waveform Graph" class="WFGraph (strict)"(error in=w1853, "Cursor Palette Vis"=FALSE ("Cursor Legend Visible")) -> (error out=w1854:errorcluster)  [unwired: 1 in, 1 out]
            n830 = invoke on="Waveform Graph" class="WFGraph (strict)" method="Get Image"(error in=w1854, "image depth"=24 ("Image Depth")) -> (error out=w1856:errorcluster, "image data"=w1855:T9)  [unwired: 4 in, 4 out]
            n831 = call <vilib>:"Write PNG File.vi"("compression (default)"=9, "error in (no error)"=w1856, "image data"=w1855) -> ("error out"=w1857:errorcluster)  [unwired: 7 in, 1 out]
            n832 = property on="Waveform Graph" class="WFGraph (strict)"(error in=w1857, "Cursor Palette Vis"=TRUE ("Cursor Legend Visible")) -> (error out=w1858:errorcluster)  [unwired: 1 in, 1 out]
            n833 = for {
              N: w1859 -> [_]
              tunnel: w1858 -> [w1863]
              i -> [w1860]
              n834 = property on="Waveform Graph" class="WFGraph (strict)"(error in=w1863, "Active Cursor"=w1860) -> (error out=w1862:errorcluster)  [unwired: 1 in, 1 out]
              n835 = property on="Waveform Graph" class="WFGraph (strict)"(error in=w1862, "Cursor.Visible"=TRUE) -> ()  [unwired: 1 in, 2 out]
            }
          }
          frame True {
            n836 = property on="Graph" class="IntGraph (strict)"() -> ("CrsrLis"=w1871:T8)  [unwired: 2 in, 2 out]
            n837 = Array Size(array=w1871) -> (size(s)=w1868:i32)
            n838 = for {
              N: w1868 -> [_]
              tunnel: [w1884] -> w1870
              i -> [w1887]
              n839 = property on="Graph" class="IntGraph (strict)"("Active Cursor"=w1887) -> (error out=w1886:errorcluster)  [unwired: 2 in, 1 out]
              n840 = property on="Graph" class="IntGraph (strict)"(error in=w1886, "Cursor.Visible"=FALSE) -> (error out=w1884:errorcluster)  [unwired: 1 in, 1 out]
            }
            n841 = property on="Graph" class="IntGraph (strict)"(error in=w1870, "Cursor Palette Vis"=FALSE ("Cursor Legend Visible")) -> (error out=w1874:errorcluster)  [unwired: 1 in, 1 out]
            n842 = invoke on="Graph" class="IntGraph (strict)" method="Get Image"(error in=w1874, "image depth"=24 ("Image Depth")) -> (error out=w1878:errorcluster, "image data"=w1879:T9)  [unwired: 4 in, 4 out]
            n843 = call <vilib>:"Write PNG File.vi"("compression (default)"=9, "error in (no error)"=w1878, "image data"=w1879) -> ("error out"=w1873:errorcluster)  [unwired: 7 in, 1 out]
            n844 = property on="Graph" class="IntGraph (strict)"(error in=w1873, "Cursor Palette Vis"=TRUE ("Cursor Legend Visible")) -> (error out=w1869:errorcluster)  [unwired: 1 in, 1 out]
            n845 = for {
              N: w1868 -> [_]
              tunnel: w1869 -> [w1880]
              i -> [w1883]
              n846 = property on="Graph" class="IntGraph (strict)"(error in=w1880, "Active Cursor"=w1883) -> (error out=w1882:errorcluster)  [unwired: 1 in, 1 out]
              n847 = property on="Graph" class="IntGraph (strict)"(error in=w1882, "Cursor.Visible"=TRUE) -> ()  [unwired: 1 in, 2 out]
            }
          }
        }
      }
    }
  }
  n848 = flat-sequence {
    tunnel: w10 -> [w1889]
    tunnel: [w1889] -> w9
    tunnel: w8 -> [_]
    frame #0 {
      n849 = local write "End"(FALSE ("End")) -> ()
    }
  }
  n850 = flat-sequence {
    tunnel: [w1891] -> w11
    tunnel: w9 -> [w1890]
    frame #0 {
      n851 = disable-structure shown="Disabled" {
        frame Disabled {
          n852 = Wait (ms)(milliseconds to wait=u32 50) -> ()  [unwired: 1 out]
        }
        frame Enabled {
        }
      }
      n853 = Unbundle By Name(w1890) -> ("reference"=w1891:refnum<visa-resource-name>)
    }
  }
  n854 = VISA Close(VISA resource name=w11) -> ()  [unwired: 1 in, 1 out]
